vi "Steuerprogramm-29-05-17.vi"() -> ()   [LabVIEW 2010]
uses:
  Emil/Licor-Steuerung/HAGAR V/Licor-Steuerung/display/GUI_Cluster_sdv.ctl
  Emil/Licor-Steuerung/HAGAR V/Licor-Steuerung/display/GUI_Cluster_Parameter.ctl
  Emil/Licor-Steuerung/HAGAR V/Licor-Steuerung/control/Licor-Commands.ctl
  Emil/Licor-Steuerung/HAGAR V/Licor-Steuerung/control/Licor-Parameter.ctl
  Emil/Licor-Steuerung/LicorLI7000/conventions/Licor-Source.ctl
  Emil/Licor-Steuerung/HAGAR V/Licor-Steuerung/control/Licor-Pump.ctl
  Emil/Licor-Steuerung/HAGAR V/Licor-Steuerung/display/GUI_Cluster_Graph.ctl
  Emil/Licor-Steuerung/HAGAR V/Licor-Steuerung/control/Licor-Sequences.ctl
  <vilib>/rvi/interface/nirviMethod/nirviMethod.xnode
  C:/Users/HAGAR-IV/Desktop/Zeugs/markus/version feb 2012/FPGA Bitfiles/pertrasgcfpga2_FPGATarget_FPGA-Programm-01_A75D3647.lvbitx
  C:/Users/HAGAR-IV/Desktop/Zeugs/Johnny/pertrasgc fpga/FPGA-Programm-01-17.vi
  <vilib>/rvi/interface/common/niFpgaNodeNameForErrorReporting.ctl
  <vilib>/rvi/errors/niLvFpgaWhatHappensToTopLevelVI.ctl
  <vilib>/rvi/interface/nirviReadWriteControl/nirviReadWriteControl.xnode
  <vilib>/rvi/interface/nirviCloseFPGA/nirviCloseFPGA.xnode
  GVProbenvol.vi
  GVZeitenZyklen.vi
  GVECDs.vi
  GVZwangs.vi
  GVMethodenwechsel.vi
  GVTrapsMachs.vi
  GVHK1Hz.vi
  GVAIs.vi
  gvbooleschRT.vi
  GVMetavariablen.vi
  GVVentilposition.vi
  GVHorstSP.vi
  GVMWHorst.vi
  GVHeizenLH.vi
  <vilib>/Utility/error.llb/Error Cluster From Error Code.vi
  <vilib>/rvi/errors/niLvFpgaAdjustHostInterfaceError.vi
  GVaktuelleTDMS.vi
  Emil/Licor-Steuerung/HAGAR V/Licor-Steuerung/control/Emulate Licor output GV.vi
  GVChroms.vi
  GVZwangsMPV.vi
  <vilib>/FPGAPlugInAG/cRIO-9114/niLvFpga_Close_cRIO-9114.vi
  NiFpgaLv.dll
  Emil/Licor-Steuerung/HAGAR V/Licor-Steuerung/Licor-Steuerung.lvlib
  Emil/Licor-Steuerung/LicorLI7000/LicorLI7000.lvlib
panel:
  in  "Methode speichern":bool
  out "ZyklusNummernGesamt":i32[](array[numeric])
  in  "veränderte Methode benutzen":bool
  in  "Methode verändern":bool
  out "ZyklusNummern":i32[](array[numeric])
  out "Big Ben, Methodenzeit, Zykluszeit0, Zykluszeit1, Zykluszeit2A, Zykluszeit2B":i32[](array[numeric])
  in  "global stop RT":bool
  in  "Methode":i32(ring) items=["Bedingsmethode", "Startmethode", "Meßmodus", "Shut-up-Methode", "Test", "HAG2 1/2", "Startmethode", "HAG2 1/2 Aufwärmen", "LicorDruckProfil1", "LicorDruckProfil2", "LicorDruckProfil0", "LicorDruckProfil3"]
  in  "Registerkarte":T1(tab)
  out "SHOK?":bool[](array[boolean])
  out "schnelle Heizungen":string[](array[string])
  out "schnelle Heizungen":dbl[](array[numeric])
  out "HorstOK?":bool[](array[boolean])
  out "AIs3OK?":bool[](array[boolean])
  out "AIs1OK?":bool[](array[boolean])
  out "AIs1":dbl[](array[numeric])
  out "AIs1":string[](array[string])
  out "AIs2":string[](array[string])
  out "AIs3":string[](array[string])
  out "AIs2":dbl[](array[numeric])
  out "AIs3":dbl[](array[numeric])
  out "Metavariablen":string[](array[string])
  out "Metavariablen":dbl[](array[numeric])
  out "MWHorst":dbl[](array[numeric])
  out "HorstRegler":string[](array[string])
  out "AIs2OK?":bool[](array[boolean])
  out "Ventilposition":i32=1 min=1 max=6 step=1
  out "MVOK?":bool[](array[boolean])
  out "Housekeeping1":cluster{dbl[], dbl[]}(graph)
  in  "Zeitachse1":i32(ring)=1 items=["Zykluszeit [s] Mod0", "Zykluszeit [s] Mod1", "Zykluszeit [s] Mod2A", "Zykluszeit [s] Mod2B"]
  in  "dargestellte Größe 1":i32(ring)=1 items=["T1-Trap1 [°C]", "T1-Trap2 [°C]", "T1-StirlingKühlkopf [°C]", "T1-PreCol1 [°C]", "T1-PreCol2 [°C]", "T1-MainCol1a [°C]", "T1-MainCol1b [°C]", "T1-MainCol2a [°C]", "T1-MainCol2b [°C]", "T1-Bronkhorst1a [°C]", "T1-Bronkhorst1b [°C]", "T1-Bronkhorst2a [°C]", "T1-Bronkhorst2b [°C]", "T1-2Pos1B [°C]", "T1-Spare9", "T1-2Pos1A [°C]", "T1-Spare10", "T1-TurboPump [°C]", "T1-StirlingPlatine [°C]", "T1-Spare5", "T1-Spare6", "T1-Spare7", "T1-Spare8", "F1-MFM1", "F1-MFM0D [mL]", "P1-HeliumHP [bara]", "P1-HeliumLP [bara]", "P1-PumpVordruck [mbara]", "TurboSpeed", "I1-MS-AC [A]", "I1-Trap1 [A]", "I1-Trap2 [A]", "T2-ECD1a", "T2-ECD1b", "T2-ECD2a", "T2-ECD2b", "T2-Col1a", "T2-Col1b", "T2-Col2a", "T2-Col2b", "T2-Spare1", "T2-Spare2", "T2-Oven_a", "T2-Oven_b", "T2-Spare3", "T2-Spare4", "T2-Spare5", "F2-MFM0", "F2-MFM2A", "F2-MFM2B", "P2-N2O_HP", "P2-N2O_LP", "P2-CO2_HP", "P2-CO2_LP", "AI-Spare1", "FL-MFM1000mL", "AI-Spare3", "AI-Spare4", "StirlingAlarm", "StirlingEmerg.", "AI-Spare7", "AI-Spare8", "AI-Spare9", "FL-MFM30mL", "T0-DC/DC5", "I0-24V_M0", "I0-48V_M1", "I0-24V_M1", "I0-28V_M2", "T0-Spare3", "T0-Spare2", "T0-Spare4", "T0-DC/DC7", "I0-20V_Laptop", "I0-28V_M1", "I0-24V_M2", "I0-12V_Licor", "T0-Spare1", "T0-Drier", "T0-Spare5", "F0-MFM0A [L]", "TL-Licor_a", "P0-Span-HP", "P0-spare1", "P0-Stickstoff-LP", "P0-Helium-LP", "P0-Cal-HP", "P0-P9Tavco[bar]", "F0-MFM0B [L]", "TL-Licor_b", "P0-Span-LP", "P0-spare2", "P0-Stickstoff-HP", "P0-Helium-HP", "P0-Cal-LP", "F0-MFM3", "TemperaturTrap1[°C]", "TemperaturTrap2[°C]", "TemperaturPreMach1[°C]", "TemperaturPreMach2[°C]", "TemperaturMainMach1[°C]", "TemperaturMainMach2[°C]", "PrC0 [bara]", "PrC0-Licor [bara]", "PrC1-Säule1 [bara]", "PrC1-Säule2 [bara]", "MFC1-Sample [ml/min]", "PrC1-BackFlush1 [bara]", "PrC1-BackFlush2 [bara]", "MFC1-Reaktant [l/min]", "MFC2A[ml/min]", "MFC2B[ml/min]", "MFC2C[ul/min]", "PrC2A[bara]", "MFC2D[ml/min]", "MFC2E[ml/min]", "PrC2B[bara]"]
  out "Housekeeping2":cluster{dbl[], dbl[]}(graph)
  in  "Zeitachse2":i32(ring)=1 items=["Zykluszeit [s] Mod0", "Zykluszeit [s] Mod1", "Zykluszeit [s] Mod2A", "Zykluszeit [s] Mod2B"]
  in  "dargestellte Größe 2":i32(ring)=1 items=["T1-Trap1 [°C]", "T1-Trap2 [°C]", "T1-StirlingKühlkopf [°C]", "T1-PreCol1 [°C]", "T1-PreCol2 [°C]", "T1-MainCol1a [°C]", "T1-MainCol1b [°C]", "T1-MainCol2a [°C]", "T1-MainCol2b [°C]", "T1-Bronkhorst1a [°C]", "T1-Bronkhorst1b [°C]", "T1-Bronkhorst2a [°C]", "T1-Bronkhorst2b [°C]", "T1-2Pos1B [°C]", "T1-Spare9", "T1-2Pos1A [°C]", "T1-Spare10", "T1-TurboPump [°C]", "T1-StirlingPlatine [°C]", "T1-Spare5", "T1-Spare6", "T1-Spare7", "T1-Spare8", "F1-MFM1", "F1-MFM0D [mL]", "P1-HeliumHP [bara]", "P1-HeliumLP [bara]", "P1-PumpVordruck [mbara]", "TurboSpeed", "I1-MS-AC [A]", "I1-Trap1 [A]", "I1-Trap2 [A]", "T2-ECD1a", "T2-ECD1b", "T2-ECD2a", "T2-ECD2b", "T2-Col1a", "T2-Col1b", "T2-Col2a", "T2-Col2b", "T2-Spare1", "T2-Spare2", "T2-Oven_a", "T2-Oven_b", "T2-Spare3", "T2-Spare4", "T2-Spare5", "F2-MFM0", "F2-MFM2A", "F2-MFM2B", "P2-N2O_HP", "P2-N2O_LP", "P2-CO2_HP", "P2-CO2_LP", "AI-Spare1", "FL-MFM1000mL", "AI-Spare3", "AI-Spare4", "StirlingAlarm", "StirlingEmerg.", "AI-Spare7", "AI-Spare8", "AI-Spare9", "FL-MFM30mL", "T0-DC/DC5", "I0-24V_M0", "I0-48V_M1", "I0-24V_M1", "I0-28V_M2", "T0-Spare3", "T0-Spare2", "T0-Spare4", "T0-DC/DC7", "I0-20V_Laptop", "I0-28V_M1", "I0-24V_M2", "I0-12V_Licor", "T0-Spare1", "T0-Drier", "T0-Spare5", "F0-MFM0A [L]", "TL-Licor_a", "P0-Span-HP", "P0-spare1", "P0-Stickstoff-LP", "P0-Helium-LP", "P0-Cal-HP", "P0-P9Tavco[bar]", "F0-MFM0B [L]", "TL-Licor_b", "P0-Span-LP", "P0-spare2", "P0-Stickstoff-HP", "P0-Helium-HP", "P0-Cal-LP", "F0-MFM3", "TemperaturTrap1[°C]", "TemperaturTrap2[°C]", "TemperaturPreMach1[°C]", "TemperaturPreMach2[°C]", "TemperaturMainMach1[°C]", "TemperaturMainMach2[°C]", "PrC0 [bara]", "PrC0-Licor [bara]", "PrC1-Säule1 [bara]", "PrC1-Säule2 [bara]", "MFC1-Sample [ml/min]", "PrC1-BackFlush1 [bara]", "PrC1-BackFlush2 [bara]", "MFC1-Reaktant [l/min]", "MFC2A[ml/min]", "MFC2B[ml/min]", "MFC2C[ul/min]", "PrC2A[bara]", "MFC2D[ml/min]", "MFC2E[ml/min]", "PrC2B[bara]"]
  out "Detektor 2":cluster{dbl[], dbl[]}[](graph)
  in  "Detektor":i32(ring) items=["ECD1", "ECD2"]
  in  "HK1YMin":dbl
  in  "HK1YMax":dbl=100.0
  in  "HK2YMin":dbl
  in  "HK2YMax":dbl=100.0
  in  "DetYMin":dbl
  in  "DetYMax":dbl=100.0
  in  "NeuerRefstrom":bool
  in  "RefStromECD1":i16 min=0 max=2500 step=1
  in  "RefStromECD2":i16 min=0 max=2500 step=1
  out "schnelleAnzeige":cluster{dbl[], dbl[]}(graph)
  in  "TafelWischen!":bool
  in  "dargestellte Größe 3":i32(ring)=1 items=["TemperaturTrap1[°C]", "TemperaturTrap2[°C]", "TemperaturPreMach1[°C]", "TemperaturPreMach2[°C]", "TemperaturMainMach1[°C]", "TemperaturMainMach2[°C]", "PrC0 [bara]", "PrC0-Licor [bara]", "PrC1-Säule1 [bara]", "PrC1-Säule2 [bara]", "MFC1-Sample [ml/min]", "PrC1-BackFlush1 [bara]", "PrC1-BackFlush2 [bara]", "MFC1-Reaktant [l/min]", "MFC2A[ml/min]", "MFC2B[ml/min]", "MFC2C[ul/min]", "PrC2A[bara]", "MFC2D[ml/min]", "MFC2E[ml/min]", "PrC2B[bara]"]
  in  "An/Aus":bool
  in  "Registerkarte 2":T2(tab)
  in  "GUI_Cluster_Graph":T3={"time (global)"=0.0, "command queue"=[], "Rohdaten"=[], "Graph"={"X"=[], "Y"=[]}, "Manuelle Steuerung"={"Sequenz"=enum."test", "Manuelle Steuerung An/Aus"=FALSE}, "Sequenz out"={"sequence"=enum."WAIT", "Zeitpunkt next"=0.0, "delta t"=0.0}} caption="Cluster" {"Sequenz out"."Zeitpunkt next" format="%<%H:%M:%S%3u>T"; "time (global)" format="%<%H:%M:%S%3u\n%m/%d/%y>T"}
  in  "GUI_Cluster_Parameter":T5={"warmup (sequence)"=[{"time"=60, "Enum"=enum."wait"}], "calibrate S (sequence)"=[{"time"=60, "Enum"=enum."wait"}, {"time"=2, "Enum"=enum."getCalibrationParameter"}, {"time"=8, "Enum"=enum."calibration-S-CO2"}, {"time"=2, "Enum"=enum."getCalibrationParameter"}], "calibrate Z (sequence)"=[{"time"=60, "Enum"=enum."wait"}, {"time"=2, "Enum"=enum."getCalibrationParameter"}, {"time"=8, "Enum"=enum."calibration-Z-H2O"}, {"time"=2, "Enum"=enum."getCalibrationParameter"}, {"time"=8, "Enum"=enum."calibration-Z-CO2"}, {"time"=2, "Enum"=enum."getCalibrationParameter"}], "initialize (sequence)"=[{"time"=30, "Enum"=enum."wait"}, {"time"=2, "Enum"=enum."setPumpSlow"}, {"time"=2, "Enum"=enum."setPumpMedium"}, {"time"=2, "Enum"=enum."setPumpFast"}, {"time"=10, "Enum"=enum."initialize"}, {"time"=4, "Enum"=enum."getCalibrationParameter"}, {"time"=2, "Enum"=enum."resetH2O"}, {"time"=4, "Enum"=enum."resetCO2"}, {"time"=4, "Enum"=enum."getCalibrationParameter"}, {"time"=2, "Enum"=enum."setZeroParameter"}, {"time"=4, "Enum"=enum."getCalibrationParameter"}, {"time"=2, "Enum"=enum."setReference"}, {"time"=4, "Enum"=enum."getLicorTime"}, {"time"=5, "Enum"=enum."getInfo"}], "Licor-parameter"={"CO2 ref"=402.3, "CO2 span"=392.3, "H2O ref"=0.0, "H2O span"=0.0, "Zi"=1.2, "Zt"=6.494e-05, "Zm"=0.0, "S"=1.34, "Temp [C]"=45.0, "Pressure [hPa]"=1013.0, "Licor-Sources"=["CO2A W", "CO2B W", "H2OA W", "H2OB W", "T C", "T V", "P kPa", "P V", "RH %", "CO2A um/m", "CO2B um/m", "H2OA mm/m", "H2OB mm/m"], "Licor-Pump"="Off", "Zeitstempel"=timestamp(0 s since 1904-01-01)}} {"Licor-parameter"."Pressure [hPa]" format="%_5g"; "Licor-parameter"."Temp [C]" format="%.2f"; "Licor-parameter"."CO2 ref" format="%.2f"; "Licor-parameter"."CO2 span" format="%.2g"; "Licor-parameter"."H2O ref" format="%.2g"; "Licor-parameter"."H2O span" format="%.2g"; "Licor-parameter"."Zt" format="%#_4g"}
  in  "GUI_Cluster_sdv":T10={"Graph_sdv"={"X"=[], "Y"=[]}, "Breite"=20, "Berechnen"=FALSE, "residue"=0.0} {"residue" format="%_6g"}
  in  "VISA resource name":refnum<visa-resource-name>="ASRL1::INSTR" caption="VISA-Ressourcenname"
  in  "ServosWarmHigh (us)KaltHigh(us)":T11={"Servo1WarmHigh(us)"=1000, "Servo1KaltHigh(us)"=1000, "Servo2WarmHigh(us)"=2030, "Servo2KaltHigh(us)"=2030}
  out "TDMSwriteECD":errorcluster
  out "AIsFIFOread":errorcluster
  out "MWTrapsMachs":errorcluster
  out "TDMSwriteHK":errorcluster
  out "TDMScloseHK":errorcluster
  out "TDMSopenHK":errorcluster
  out "TDMScloseECD2":errorcluster
  out "TDMSopenECD2":errorcluster
  out "TDMScloseECD1":errorcluster
  out "TDMSopenECD1":errorcluster
  out "FIFOwriteRS485":errorcluster
  out "SerielleKomm.":errorcluster
  out "LH":errorcluster
  out "Zyklus":errorcluster
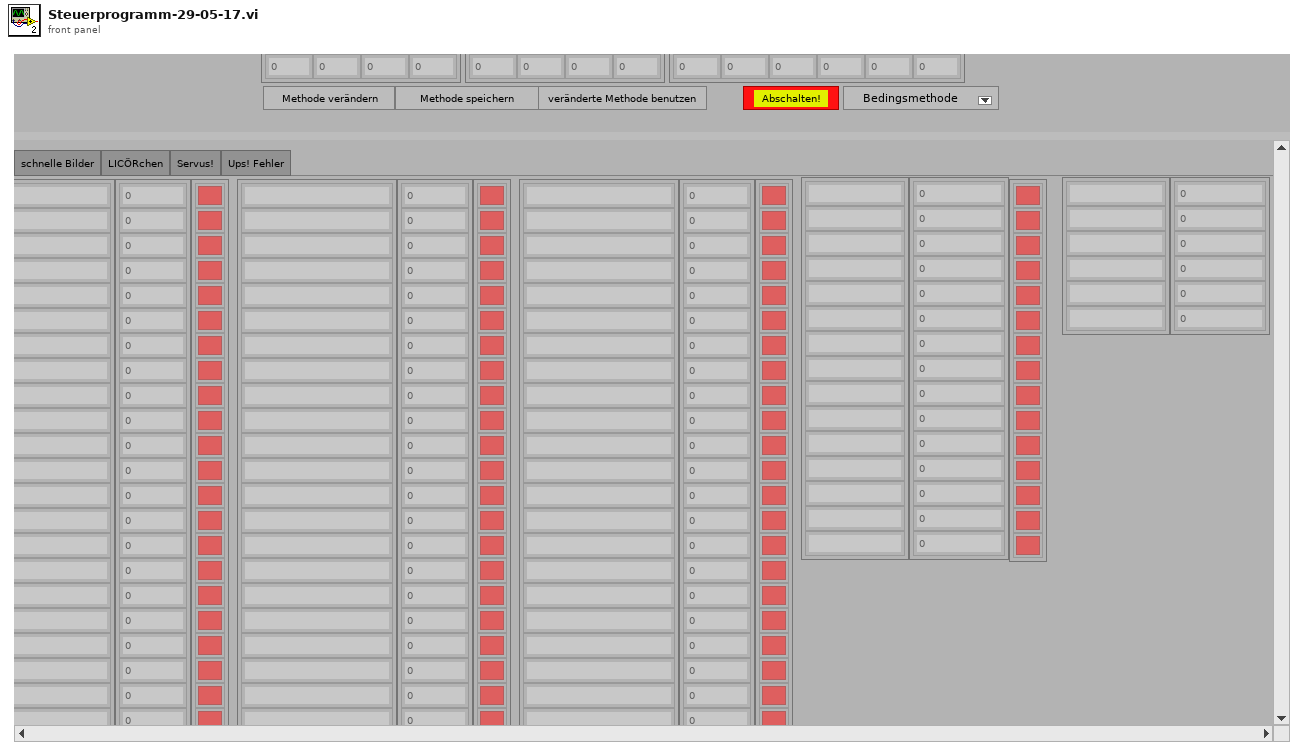
[diagram p1: front panel]
types:
  T1 = enum32{"Tabellen", "Bilder", "schnelle Bilder", "LICÖRchen", "Servus!", "Ups! Fehler"}
  T2 = enum32{"Graph", "Parameter / Sequenzen", "sdv", "debug"}
  T3 = typedef "Licor-Steuerung.lvlib/GUI_Cluster_Graph.ctl" = cluster{"time (global)":dbl, "command queue":cluster{"Zeit [s]":i32, "Befehl":string}[], "Rohdaten":string[], "Graph":cluster{"X":dbl[], "Y":dbl[]}, "Manuelle Steuerung":cluster{"Sequenz":T4, "Manuelle Steuerung An/Aus":bool}, "Sequenz out":cluster{"sequence":T4, "Zeitpunkt next":dbl, "delta t":dbl}}
  T4 = typedef "Licor-Steuerung.lvlib/Licor-Sequences.ctl" = enum16{"test", "WAIT", "warmup", "initialize", "calibrate Z", "calibrate S"}
  T5 = typedef "Licor-Steuerung.lvlib/GUI_Cluster_Parameter.ctl" = cluster{"warmup (sequence)":cluster{"time":i32, "Enum":T6}[], "calibrate S (sequence)":cluster{"time":i32, "Enum":T6}[], "calibrate Z (sequence)":cluster{"time":i32, "Enum":T6}[], "initialize (sequence)":cluster{"time":i32, "Enum":T6}[], "Licor-parameter":T7}
  T6 = typedef "Licor-Steuerung.lvlib/Licor-Commands.ctl" = enum16{"wait", "initialize", "resetCO2", "resetH2O", "getReference", "setReference", "calibration-Z-CO2", "calibration-Z-H2O", "calibration-S-CO2", "calibration-S-H2O", "getCalibrationParameter", "setZeroParameter", "setLicorTime", "getLicorTime", "setPumpFlowrate", "setPumpSlow", "setPumpMedium", "setPumpFast", "getInfo"}
  T7 = typedef "Licor-Steuerung.lvlib/Licor-Parameter.ctl" = cluster{"CO2 ref":dbl, "CO2 span":dbl, "H2O ref":dbl, "H2O span":dbl, "Zi":dbl, "Zt":dbl, "Zm":dbl, "S":dbl, "Temp [C]":dbl, "Pressure [hPa]":dbl, "Licor-Sources":T8[], "Licor-Pump":T9, "Zeitstempel":timestamp}
  T8 = typedef "LicorLI7000.lvlib/Licor-Source.ctl" = string
  T9 = typedef "Licor-Steuerung.lvlib/Licor-Pump.ctl" = string
  T10 = typedef "Licor-Steuerung.lvlib/GUI_Cluster_sdv.ctl" = cluster{"Graph_sdv":cluster{"X":dbl[], "Y":dbl[]}, "Breite":i32, "Berechnen":bool, "residue":dbl}
  T11 = cluster{"Servo1WarmHigh(us)":u32, "Servo1KaltHigh(us)":u32, "Servo2WarmHigh(us)":u32, "Servo2KaltHigh(us)":u32}
  T12 = cluster{"DIOsMod0Nr":i32[], "DIOsMod1Nr":i32[], "DIOsMod2ANr":i32[], "DIOsMod2BNr":i32[], "AIsLH":i32[], "AnzahlRegler/Modul":i32[], "Regler für den Probenfluß":i32, "SPvorgebenMod0":string[], "SPvorgebenMod1":string[], "SPvorgebenMod2A":string[], "SPvorgebenMod2B":string[], "MWAntwortMod0":string[], "MWAntwortMod1":string[], "MWAntwortMod2A":string[], "MWAntwortMod2B":string[], "FaktorMod0":dbl[], "FaktorMod1":dbl[], "FaktorMod2A":dbl[], "FaktorMod2B":dbl[], "MWabfragenMod0":string[], "MWabfragenMod1":string[], "MWabfragenMod2A":string[], "MWabfragenMod2B":string[], "Modul1/AI koeff":dbl[][], "Modul2/AI koeff":dbl[][], "Modul3/AI koeff":dbl[][], "Traps/MachsKoeff":dbl[][], "Modul1/AIsNamen":string[], "Modul2/AIsNamen":string[], "Modul3/AIsNamen":string[], "DIOsMod0Name":string[], "DIOsMod1Name":string[], "DIOsMod2AName":string[], "DIOsMod2BName":string[], "ReglerNameMod0":string[], "ReglerNameMod1":string[], "ReglerNameMod2A":string[], "ReglerNameMod2B":string[], "Startmethode":i32, "Dateiordner Housekeeping":path, "Dateiname Housekeeping":string, "DateiordnerECD1":path, "DateinameECD1":string, "DateiordnerECD2":path, "DateinameECD2":string, "LangsameHeizungen":string[], "ModuleLH":i32[], "Metavariablen":string[], "Modul1/AI sicherer Bereich":dbl[][], "Modul2/AI sicherer Bereich":dbl[][], "Modul3/AI sicherer Bereich":dbl[][], "Traps/Machs sicherer Bereich":dbl[][], "ReglerMod0 sicherer Bereich":dbl[][], "ReglerMod1 sicherer Bereich":dbl[][], "ReglerMod2A sicherer Bereich":dbl[][], "ReglerMod2B sicherer Bereich":dbl[][], "Metavariablen grüner Bereich":dbl[][]}
  T13 = cluster{"Zykluslängen [s]":dbl[], "ZeitpktDIOsMod0":dbl[], "ZeitpktDIOsMod1":dbl[], "ZeitpktDIOsMod2A":dbl[], "ZeitpktDIOsMod2B":dbl[], "DIOsSPMod0":bool[][], "DIOsSPMod1":bool[][], "DIOsSPMod2A":bool[][], "DIOsSPMod2B":bool[][], "Mod0HorstZeitpkt":dbl[], "Mod1HorstZeitpkt":dbl[], "Mod2AHorstZeitpkt":dbl[], "Mod2BHorstZeitpkt":dbl[], "HorstSPMod0":dbl[][], "HorstSPMod1":dbl[][], "HorstSPMod2A":dbl[][], "HorstSPMod2B":dbl[][], "LHSetpoints":dbl[], "LHHeizen?":bool[], "ZPktFPGABoolesch":dbl[], "FPGABoolesch":bool[][], "ZeitpktFPGAPID":dbl[], "FPGAPID":cluster{"proportional gain (Kc)":fxp<+/-,16,8>, "integral gain (Kc*Ts/Ti)":fxp<+/-,16,8>, "derivative gain (Kc*Td/Ts)":fxp<+/-,16,8>}[][], "ZeitpktFPGAFixp":dbl[], "SHSetpoints":dbl[][], "t_PreMach1":dbl[], "T_PreMach1":dbl[], "t_PreMach2":dbl[], "T_PreMach2":dbl[], "PIDs für \"träge\" Heizungen":cluster{"proportional gain (Kc)":dbl, "integral time (Ti, min)":dbl, "derivative time (Td, min)":dbl}[], "Zwangsbedingungen":dbl[][], "Dateien fürs MS schicken?":bool, "ZeitpunkteMPV":dbl[], "SPMPV":i32[], "ZeitpktMS-1":dbl, "ZeitpktMS-2":dbl, "Int.Start1":dbl, "Int.Stop1":dbl, "Int.Start2":dbl, "Int.Stop2":dbl, "Methodenname":string, "t_MainMach1":dbl[], "T_MainMach1":dbl[], "t_MainMach2":dbl[], "T_MainMach2":dbl[]}[]
  T14 = enum16{"open", "replace", "create", "open or create", "replace or create", "replace or create with confirmation"}
  T15 = typedef "niFpgaNodeNameForErrorReporting.ctl" = enum16{"Open FPGA VI Reference", "Read/Write Control", "Invoke Method: Abort", "Invoke Method: Acknowledge IRQ", "Invoke Method: Download", "Invoke Method: FIFO.Configure", "Invoke Method: FIFO.Read", "Invoke Method: FIFO.Start", "Invoke Method: FIFO.Stop", "Invoke Method: FIFO.Write", "Invoke Method: Reset", "Invoke Method: Run", "Invoke Method: Wait on IRQ", "Close FPGA VI Reference"}
  T16 = typedef "niLvFpgaWhatHappensToTopLevelVI.ctl" = enum16{"top level VI scripted behind XNode", "top level VI inlined behind XNode"}
  T17 = cluster{"Zyklus1":i32, "Zeitachse1":i32, "dargestellte Größe 1":i32, "Zyklus2":i32, "Zeitachse2":i32, "dargestellte Größe 2":i32}
  T18 = cluster{"DIOsMod0Name":string[], "DIOsMod1Name":string[], "DIOsMod2AName":string[], "DIOsMod2BName":string[], "ReglerNameMod0":string[], "ReglerNameMod1":string[], "ReglerNameMod2A":string[], "ReglerNameMod2B":string[], "LangsameHeizungen":string[]}
  T19 = cluster{"Zykluslängen [s]":dbl[], "ZeitpktDIOsMod0":dbl[], "ZeitpktDIOsMod1":dbl[], "ZeitpktDIOsMod2A":dbl[], "ZeitpktDIOsMod2B":dbl[], "DIOsSPMod0":bool[][], "DIOsSPMod1":bool[][], "DIOsSPMod2A":bool[][], "DIOsSPMod2B":bool[][], "Mod0HorstZeitpkt":dbl[], "Mod1HorstZeitpkt":dbl[], "Mod2AHorstZeitpkt":dbl[], "Mod2BHorstZeitpkt":dbl[], "HorstSPMod0":dbl[][], "HorstSPMod1":dbl[][], "HorstSPMod2A":dbl[][], "HorstSPMod2B":dbl[][], "LHSetpoints":dbl[], "LHHeizen?":bool[], "ZPktFPGABoolesch":dbl[], "FPGABoolesch":bool[][], "ZeitpktFPGAPID":dbl[], "FPGAPID":cluster{"proportional gain (Kc)":fxp<+/-,16,8>, "integral gain (Kc*Ts/Ti)":fxp<+/-,16,8>, "derivative gain (Kc*Td/Ts)":fxp<+/-,16,8>}[][], "ZeitpktFPGAFixp":dbl[], "SHSetpoints":dbl[][], "t_PreMach1":dbl[], "T_PreMach1":dbl[], "t_PreMach2":dbl[], "T_PreMach2":dbl[], "PIDs für \"träge\" Heizungen":cluster{"proportional gain (Kc)":dbl, "integral time (Ti, min)":dbl, "derivative time (Td, min)":dbl}[], "Zwangsbedingungen":dbl[][], "Dateien fürs MS schicken?":bool, "ZeitpunkteMPV":dbl[], "SPMPV":i32[], "ZeitpktMS-1":dbl, "ZeitpktMS-2":dbl, "Int.Start1":dbl, "Int.Stop1":dbl, "Int.Start2":dbl, "Int.Stop2":dbl, "Methodenname":string, "t_MainMach1":dbl[], "T_MainMach1":dbl[], "t_MainMach2":dbl[], "T_MainMach2":dbl[]}
  T20 = cluster{"Modul1/AI sicherer Bereich":dbl[][], "Modul2/AI sicherer Bereich":dbl[][], "Modul3/AI sicherer Bereich":dbl[][], "Traps/Machs sicherer Bereich":dbl[][], dbl[][], "Metavariablen grüner Bereich":dbl[][]}
  T21 = cluster{"created path":path, "created path":path, "created path":path, "Dateiname Housekeeping":string, "DateinameECD1":string, "DateinameECD2":string, "tdms0":refnum<k34>, "tdms1":refnum<k34>, "tdms0":refnum<k34>, "tdms1":refnum<k34>, "tdms0":refnum<k34>, "tdms1":refnum<k34>}
  T22 = cluster{"proportional gain (Kc)":fxp<+/-,16,8>, "integral gain (Kc*Ts/Ti)":fxp<+/-,16,8>, "derivative gain (Kc*Td/Ts)":fxp<+/-,16,8>}[][]
  T23 = cluster{"proportional gain (Kc)":dbl, "integral time (Ti, min)":dbl, "derivative time (Td, min)":dbl}[]
  T24 = cluster{cluster{"ZeitpktDIOsMod2B":dbl[]}[], cluster{"DIOsSPMod2B":bool[][]}[], cluster{"Mod2BHorstZeitpkt":dbl[]}[], cluster{"HorstSPMod2B":dbl[][]}[], "LHHeizen?":bool[], "ZPktFPGABoolesch":dbl[], "FPGABoolesch":bool[][], "ZeitpktFPGAPID":dbl[], "FPGAPID":cluster{"proportional gain (Kc)":fxp<+/-,16,8>, "integral gain (Kc*Ts/Ti)":fxp<+/-,16,8>, "derivative gain (Kc*Td/Ts)":fxp<+/-,16,8>}[][], "ZeitpktFPGAFixp":dbl[], "SHSetpoints":dbl[][], "t_PreMach1":dbl[], "T_PreMach1":dbl[], "t_PreMach2":dbl[], "T_PreMach2":dbl[], "ZeitpunkteMPV":dbl[], "SPMPV":i32[], "t_MainMach1":dbl[], "T_MainMach1":dbl[], "t_MainMach2":dbl[], "T_MainMach2":dbl[]}
  T25 = cluster{"Zykluslängen [s]":dbl[], "ZeitpktDIOsMod0":dbl[], "ZeitpktDIOsMod1":dbl[], "ZeitpktDIOsMod2A":dbl[], "ZeitpktDIOsMod2B":dbl[], "DIOsSPMod0":bool[][], "DIOsSPMod1":bool[][], "DIOsSPMod2A":bool[][], "DIOsSPMod2B":bool[][], "Mod0HorstZeitpkt":dbl[], "Mod1HorstZeitpkt":dbl[], "Mod2AHorstZeitpkt":dbl[], "Mod2BHorstZeitpkt":dbl[], "HorstSPMod0":dbl[][], "HorstSPMod1":dbl[][], "HorstSPMod2A":dbl[][], "HorstSPMod2B":dbl[][], "LangsameHeizungenSP":dbl[], "LHHeizen?":bool[], "ZPktFPGABoolesch":dbl[], "FPGABoolesch":bool[][], "ZeitpktFPGAPID":dbl[], "FPGAPID":cluster{"proportional gain (Kc)":fxp<+/-,16,8>, "integral gain (Kc*Ts/Ti)":fxp<+/-,16,8>, "derivative gain (Kc*Td/Ts)":fxp<+/-,16,8>}[][], "ZeitpktFPGAFixp":dbl[], "FPGAFixp":dbl[][], "t_PreMach1":dbl[], "T_PreMach1":dbl[], "t_PreMach2":dbl[], "T_PreMach2":dbl[], "PIDs für \"träge\" Heizungen":cluster{"proportional gain (Kc)":dbl, "integral time (Ti, min)":dbl, "derivative time (Td, min)":dbl}[], "Zwangsbedingungen":dbl[][], "MS-Daten?":bool, "ZeitpunkteMPV":dbl[], "SetpointMPV":i32[], "ZeitpktMS-1":dbl, "ZeitpktMS-2":dbl, "Int.Start1":dbl, "Int.Stop1":dbl, "Int.Start2":dbl, "Int.Stop2":dbl, "Methodenname":string, "t_MainMach1":dbl[], "T_MainMach1":dbl[], "t_MainMach2":dbl[], "T_MainMach2":dbl[]}
  T26 = cluster{"ZyklusNummern":i32[], "ZeilennummernDIOs":i32[], "ZwangsDIO?":cluster{bool[]}[], "ZeilennummernHorst":i32[], "ZwangsHorst?":cluster{bool[]}[], "ZeileFPGABoolesch":i32, "ZwangsFPGABoolesch?":bool[], "ZeileFPGAPID":i32, "ZeileFPGAFixp":i32, "ZeilePreMach1":i32, "ZeilePreMach2":i32, "ZeilennummerMPV":i32, "ZeileMainMach1":i32, "ZeileMainMach2":i32, "ZwangsMPV?":bool}
  T27 = cluster{"ZyklusNummern":i32[], i32[], "ZwangsDIO?":cluster{bool[]}[], i32[], "ZwangsHorst?":cluster{bool[]}[], i32, "ZwangsFPGABoolesch?":bool[], i32, i32, "ZeileMach":i32, "ZeileMach":i32, i32, "ZeileMach":i32, "ZeileMach":i32, "ZwangsMPV?":bool}
  T28 = cluster{string[], string[], string[], dbl[], dbl[], dbl[]}
  T29 = cluster{"Befehle1":string[], "Befehle2":string[], "Befehle3":string[]}
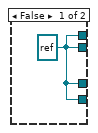
[diagram p2: hidden frame]
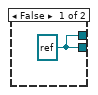
[diagram p3: hidden frame]
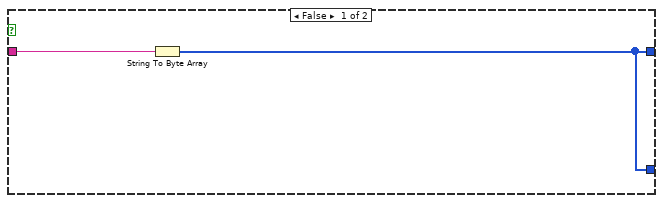
[diagram p6: hidden frame]
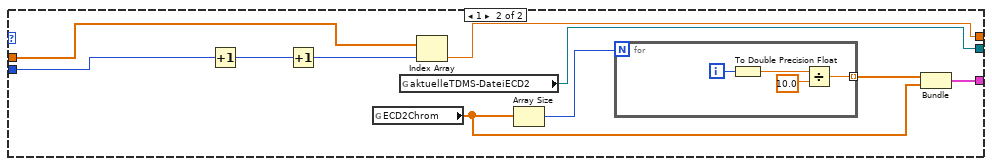
[diagram p13: hidden frame]
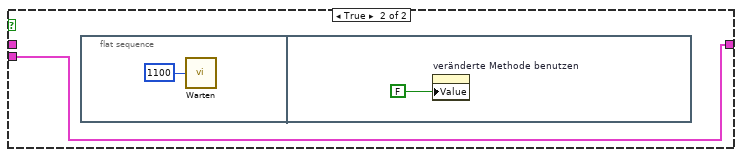
[diagram p14: hidden frame]
diagram:
  n1 = Open/Create/Replace File(file path (use dialog)=path "c:/einstellungen.perx" ("Datei (Dialog verwenden)"), operation (0:open)=T14."open" ("Operation (0:Öffnen)")) -> (refnum out=w13:refnum<file>)  [unwired: 4 in, 2 out]
  n2 = Open/Create/Replace File(file path (use dialog)=path "c:/methoden.per" ("Datei (Dialog verwenden)"), operation (0:open)=T14."open" ("Operation (0:Öffnen)")) -> (refnum out=w8:refnum<file>)  [unwired: 4 in, 2 out]
  n3 = Read from Binary File(5:T12 {"DIOsMod0Nr"=[], "DIOsMod1Nr"=[], "DIOsMod2ANr"=[], "DIOsMod2BNr"=[], "AIsLH"=[], "AnzahlRegler/Modul"=[], "Regler für den Probenfluß"=0, "SPvorgebenMod0"=[], "SPvorgebenMod1"=[], "SPvorgebenMod2A"=[], "SPvorgebenMod2B"=[], "MWAntwortMod0"=[], "MWAntwortMod1"=[], "MWAntwortMod2A"=[], "MWAntwortMod2B"=[], "FaktorMod0"=[], "FaktorMod1"=[], "FaktorMod2A"=[], "FaktorMod2B"=[], "MWabfragenMod0"=[], "MWabfragenMod1"=[], "MWabfragenMod2A"=[], "MWabfragenMod2B"=[], "Modul1/AI koeff"=[], "Modul2/AI koeff"=[], "Modul3/AI koeff"=[], "Traps/MachsKoeff"=[], "Modul1/AIsNamen"=[], "Modul2/AIsNamen"=[], "Modul3/AIsNamen"=[], "DIOsMod0Name"=[], "DIOsMod1Name"=[], "DIOsMod2AName"=[], "DIOsMod2BName"=[], "ReglerNameMod0"=[], "ReglerNameMod1"=[], "ReglerNameMod2A"=[], "ReglerNameMod2B"=[], "Startmethode"=0, "Dateiordner Housekeeping"=path "", "Dateiname Housekeeping"="", "DateiordnerECD1"=path "", "DateinameECD1"="", "DateiordnerECD2"=path "", "DateinameECD2"="", "LangsameHeizungen"=[], "ModuleLH"=[], "Metavariablen"=[], "Modul1/AI sicherer Bereich"=[], "Modul2/AI sicherer Bereich"=[], "Modul3/AI sicherer Bereich"=[], "Traps/Machs sicherer Bereich"=[], "ReglerMod0 sicherer Bereich"=[], "ReglerMod1 sicherer Bereich"=[], "ReglerMod2A sicherer Bereich"=[], "ReglerMod2B sicherer Bereich"=[], "Metavariablen grüner Bereich"=[]} ("output cluster"), 11:w13) -> (2:w11:T12, 3:w12:refnum<file>)  [unwired: 4 in, 2 out]
  n4 = Read from Binary File(5:T13 [], 11:w8) -> (2:w6:T13, 3:w7:refnum<file>)  [unwired: 4 in, 2 out]
  n5 = Close File(refnum=w12) -> ()  [unwired: 1 in, 2 out]
  n6 = Close File(refnum=w7) -> ()  [unwired: 1 in, 2 out]
  n7 = flat-sequence {
    tunnel: [w55] -> w41
    tunnel: [w112] -> w40
    tunnel: [w59] -> w38
    tunnel: [w246] -> w37
    tunnel: [w248] -> w36
    tunnel: [w240] -> w35
    tunnel: [w247] -> w34
    tunnel: [w170] -> w33
    tunnel: [w239] -> w32
    tunnel: [w238] -> w31
    tunnel: [w232] -> w30
    tunnel: [w173] -> w29
    tunnel: [w147] -> w28
    tunnel: [w245] -> w27
    tunnel: [w237] -> w26
    tunnel: [w236] -> w25
    tunnel: [w228] -> w24
    tunnel: [w227] -> w23
    tunnel: [w226] -> w22
    tunnel: [w225] -> w21
    tunnel: [w224] -> w20
    tunnel: [w223] -> w19
    tunnel: [w220] -> w18
    tunnel: [w202] -> w17
    tunnel: w11 -> [w88]
    tunnel: [w201] -> w16
    tunnel: w6 -> [w113]
    tunnel: [w112] -> w5
    tunnel: [w88] -> w3
    tunnel: [w50] -> w1
    tunnel: w41 -> [w445]
    tunnel: w40 -> [w518]
    tunnel: [w445] -> w39
    tunnel: w38 -> [_]
    tunnel: w37 -> [w476]
    tunnel: w36 -> [w475]
    tunnel: w35 -> [w477]
    tunnel: w34 -> [w474]
    tunnel: w33 -> [w449]
    tunnel: w32 -> [w444]
    tunnel: w31 -> [w441]
    tunnel: w30 -> [w438]
    tunnel: w29 -> [w439]
    tunnel: w28 -> [w442]
    tunnel: w27 -> [w516]
    tunnel: w26 -> [w447]
    tunnel: w25 -> [w517]
    tunnel: w24 -> [w420]
    tunnel: w23 -> [w419]
    tunnel: w22 -> [w418]
    tunnel: w21 -> [w514]
    tunnel: w20 -> [w513]
    tunnel: w19 -> [w512]
    tunnel: w18 -> [w466]
    tunnel: w17 -> [w448]
    tunnel: w16 -> [w437]
    tunnel: w6 -> [w436]
    tunnel: w5 -> [w434]
    tunnel: w3 -> [_]
    tunnel: w1 -> [w413]
    tunnel: w39 -> [w1355]
    frame #0 {
      w114 = TRUE
      w129 = 0.0 ("Probenvol.1")
      w136 = dbl[] [-1.0] ("ECD1MW")
      w137 = FALSE ("ECD1Empfangen?")
      w128 = string[] ["TemperaturTrap1[°C]", "TemperaturTrap2[°C]", "TemperaturPreMach1[°C]", "TemperaturPreMach2[°C]", "TemperaturMainMach1[°C]", "TemperaturMainMach2[°C]"]
      w243 = string[] ["Big Ben [s]", "Methodenzeit [s]", "Zykluszeit [s] Mod0", "Zykluszeit [s] Mod1", "Zykluszeit [s] Mod2A", "Zykluszeit [s] Mod2B"]
      w233 = FALSE ("Undefinierte Werte möglich")
      w234 = FALSE ("global stop RT")
      n8 = for {
        tunnel: [w408] -> w241 mode=indexing
        tunnel: w113 -> [w409] mode=indexing
        n9 = Unbundle(w409) -> ("Methodenname"=w408:string)  [unwired: 44 out]
      }
      n10 = Unbundle(w88) -> ("DIOsMod0Nr"=w157:i32[], "DIOsMod1Nr"=w156:i32[], "DIOsMod2ANr"=w155:i32[], "DIOsMod2BNr"=w154:i32[], "AIsLH"=w144:i32[], "AnzahlRegler/Modul"=w147:i32[], "Regler für den Probenfluß"=w201:i32, "SPvorgebenMod0"=w200:string[], "SPvorgebenMod1"=w199:string[], "SPvorgebenMod2A"=w198:string[], "SPvorgebenMod2B"=w197:string[], "MWAntwortMod0"=w196:string[], "MWAntwortMod1"=w195:string[], "MWAntwortMod2A"=w194:string[], "MWAntwortMod2B"=w193:string[], "FaktorMod0"=w192:dbl[], "FaktorMod1"=w191:dbl[], "FaktorMod2A"=w190:dbl[], "FaktorMod2B"=w189:dbl[], "MWabfragenMod0"=w188:string[], "MWabfragenMod1"=w187:string[], "MWabfragenMod2A"=w186:string[], "MWabfragenMod2B"=w185:string[], "Modul1/AI koeff"=w184:dbl[][], "Modul2/AI koeff"=w183:dbl[][], "Modul3/AI koeff"=w182:dbl[][], "Traps/MachsKoeff"=w181:dbl[][], "Modul1/AIsNamen"=w180:string[], "Modul2/AIsNamen"=w179:string[], "Modul3/AIsNamen"=w178:string[], "DIOsMod0Name"=w86:string[], "DIOsMod1Name"=w87:string[], "DIOsMod2AName"=w85:string[], "DIOsMod2BName"=w84:string[], "ReglerNameMod0"=w103:string[], "ReglerNameMod1"=w102:string[], "ReglerNameMod2A"=w101:string[], "ReglerNameMod2B"=w100:string[], "Startmethode"=w112:i32, "Dateiordner Housekeeping"=w83:path, "Dateiname Housekeeping"=w177:string, "DateiordnerECD1"=w97:path, "DateinameECD1"=w176:string, "DateiordnerECD2"=w96:path, "DateinameECD2"=w175:string, "LangsameHeizungen"=w174:string[], "ModuleLH"=w169:i32[], "Metavariablen"=w107:string[], "Modul1/AI sicherer Bereich"=w54:dbl[][], "Modul2/AI sicherer Bereich"=w53:dbl[][], "Modul3/AI sicherer Bereich"=w52:dbl[][], "Traps/Machs sicherer Bereich"=w51:dbl[][], "ReglerMod0 sicherer Bereich"=w49:dbl[][], "ReglerMod1 sicherer Bereich"=w48:dbl[][], "ReglerMod2A sicherer Bereich"=w47:dbl[][], "ReglerMod2B sicherer Bereich"=w46:dbl[][], "Metavariablen grüner Bereich"=w44:dbl[][])
      "Metavariablen" <- w107
      n11 = Initialize Array(0, 4 ("Dimension")) -> (w130:i32[])
      n12 = Initialize Array(0.0 ("Element"), 6 ("Dimension")) -> (w133:dbl[])
      n13 = global write "GVMethodenwechsel.vi" "Methodenwechsel?"(FALSE ("Methodenwechsel?")) -> ()
      n14 = local write "NeuerRefstrom"(FALSE ("NeuerRefstrom")) -> ()
      n15 = global write "GVProbenvol.vi" "Probenvol.1"(w129) -> ()
      n16 = global write "GVProbenvol.vi" "Probenvol.2"(w129) -> ()
      n17 = global write "GVECDs.vi" "ECD1MW"(w136) -> ()
      n18 = global write "GVECDs.vi" "ECD2MW"(w136) -> ()
      n19 = global write "GVECDs.vi" "ECD1Empfangen?"(w137) -> ()
      n20 = global write "GVECDs.vi" "ECD2Empfangen?"(w137) -> ()
      n21 = property on="dargestellte Größe 2" class="Ring (strict)"("AllowUndefVals"=w233) -> ()  [unwired: 2 in, 2 out]
      n22 = property on="Zeitachse2" class="Ring (strict)"("AllowUndefVals"=w233) -> ()  [unwired: 2 in, 2 out]
      n23 = property on="Zeitachse1" class="Ring (strict)"("AllowUndefVals"=w233) -> ()  [unwired: 2 in, 2 out]
      n24 = property on="dargestellte Größe 1" class="Ring (strict)"("AllowUndefVals"=w233) -> ()  [unwired: 2 in, 2 out]
      n25 = property on="Methode" class="Ring (strict)"("AllowUndefVals"=w233) -> ()  [unwired: 2 in, 2 out]
      n26 = local write "global stop RT"(w234) -> ()
      n27 = global write "gvbooleschRT.vi" "global stop RT"(w234) -> ()
      n28 = global write "GVZeitenZyklen.vi" "ZyklusNummern"(w130) -> ()
      n29 = global write "GVZeitenZyklen.vi" "ZyklusNummernGesamt"(w130) -> ()
      n30 = global write "GVZeitenZyklen.vi" "Big Ben, Methodenzeit, Zykluszeit0, Zykluszeit1, Zykluszeit2A, Zykluszeit2B"(w133) -> ()
      n31 = property on="Methode" class="Ring (strict)"("Value"=w112) -> ()  [unwired: 2 in, 2 out]
      n32 = Initialize Array(-1.0 ("Element"), 6 ("Dimension")) -> (w140:dbl[])
      n33 = Initialize Array(FALSE, 10 ("Dimension")) -> (w148:bool[])
      n34 = Initialize Array(-1.0 ("Element"), 96 ("Dimension")) -> (w141:dbl[])
      n35 = global write "GVZwangs.vi" "ZwangsFPGABoolesch!"(w148) -> ()
      n36 = global write "GVZwangs.vi" "ZwangsFPGABoolesch?"(w148) -> ()
      n37 = global write "GVTrapsMachs.vi" "Traps/Machs"(w140) -> ()
      n38 = global write "GVAIs.vi" "AIs"(w141) -> ()
      n39 = for {
        tunnel: w147 -> [w386] mode=indexing
        tunnel: [w383] -> w146 mode=indexing
        tunnel: [w381] -> w145 mode=indexing
        n40 = Initialize Array(0.0 ("Element"), w386) -> (w384:dbl[])
        n41 = Initialize Array(FALSE, w386) -> (w382:bool[])
        n42 = Bundle(w384) -> (w383:cluster{dbl[]})  [unwired: 1 in]
        n43 = Bundle(w382) -> (w381:cluster{bool[]})  [unwired: 1 in]
      }
      n44 = Bundle("DIOsMod0Name"=w86, "DIOsMod1Name"=w87, "DIOsMod2AName"=w85, "DIOsMod2BName"=w84, "ReglerNameMod0"=w103, "ReglerNameMod1"=w102, "ReglerNameMod2A"=w101, "ReglerNameMod2B"=w100, "LangsameHeizungen"=w174) -> (w236:T18)  [unwired: 1 in]
      n45 = Build Array (concatenate)(w103, w102, w101, w100) -> (w127:string[])
      n46 = Build Array (concatenate)(w196, w195, w194, w193) -> (w247:string[])
      n47 = Build Array (concatenate)(w200, w199, w198, w197) -> (w248:string[])
      n48 = Build Array (concatenate)(w192, w191, w190, w189) -> (w240:dbl[])
      n49 = Build Array (concatenate)(w188, w187, w186, w185) -> (w246:string[])
      n50 = Build Array (concatenate)(w103, w102, w101, w100) -> (→"HorstRegler":string[])
      n51 = Build Array (concatenate)(w49, w48, w47, w46) -> (w45:dbl[][])
      n52 = Array Size(array=w107) -> (size(s)=w106:i32)
      n53 = Build Array(w157, w156, w155, w154) -> (w153:i32[][])
      n54 = Array Size(array=w174) -> (size(s)=w173:i32)
      n55 = Add Array Elements(numeric array=w147) -> (sum=w232:i32)
      n56 = Array Size(array=w144) -> (size(s)=w143:i32)
      n57 = Index Array(array=w113, index=w112) -> (element=w111:T19)
      n58 = Add Array Elements(numeric array=w147) -> (sum=w159:i32)
      n59 = Decrement(x=w169) -> (x-1=w168:i32[])
      n60 = Build Cluster Array(w157, w156, w155, w154) -> (w239:cluster{"DIOsMod2BNr":i32[]}[])
      n61 = Build Array (concatenate)(w180, w179, w178) -> (w118:string[])
      n62 = Index Array(array=w181, index (col)=2 ("Deaktivierter Index (Spalte)")) -> (element=w228:dbl[])  [unwired: 1 in]
      n63 = Index Array(array=w181, index (col)=0 ("Deaktivierter Index (Spalte)")) -> (element=w226:dbl[])  [unwired: 1 in]
      n64 = Index Array(array=w181, index (col)=1 ("Deaktivierter Index (Spalte)")) -> (element=w227:dbl[])  [unwired: 1 in]
      n65 = Concatenate Strings("?SE0,SETP,1700" ("string"), "\r\n") -> (w61:string)
      n66 = Concatenate Strings("?SE0,SETP,1100" ("string"), "\r\n") -> (w68:string)
      n67 = for {
        tunnel: w239 -> [w411] mode=indexing
        tunnel: [w412] -> w238 mode=indexing
        n68 = Unbundle(w411) -> ("DIOsMod2BNr"=w410:i32[])
        n69 = Array Size(array=w410) -> (size(s)=w412:i32)
      }
      n70 = property on="Methode" class="Ring (strict)"("Strings []"=w241) -> ()  [unwired: 2 in, 2 out]
      n71 = Bundle("Modul1/AI sicherer Bereich"=w54, "Modul2/AI sicherer Bereich"=w53, "Modul3/AI sicherer Bereich"=w52, "Traps/Machs sicherer Bereich"=w51, w45, "Metavariablen grüner Bereich"=w44) -> (w50:T20)  [unwired: 1 in]
      n72 = Build Array (concatenate)(w141, w140) -> (w139:dbl[])
      n73 = Array Size(array=w153) -> (size(s)=w152:i32[])
      n74 = Unbundle(w111) -> ("SPMPV"=w110:i32[])  [unwired: 44 out]
      n75 = Open/Create/Replace File(file path (use dialog)=path "c:/fromcriordy.txt" ("Dateipfad (Dialog verwenden)"), operation (0:open)=T14."replace or create" ("Operation (0:Öffnen)")) -> (refnum out=w205:refnum<file>, error out=w206:errorcluster)  [unwired: 4 in, 1 out]
      n76 = Initialize Array(0.0 ("element"), w106) -> (w104:dbl[])
      n77 = Initialize Array(0.0 ("Element"), w159) -> (w158:dbl[])
      n78 = Get Date/Time In Seconds() -> (seconds since 1Jan1904=w98:timestamp)
      n79 = Initialize Array(FALSE, w143) -> (w138:bool[])
      n80 = Multiply(x=w168, y=32) -> (x*y=w171:i32[])
      n81 = Initialize Array(-1.0, w159) -> (w161:dbl[])
      n82 = Array Subset(array=w118, index=32 ("Index"), length=32 ("Länge")) -> (→"AIs2":string[])
      n83 = Array Subset(array=w118, index=0 ("Index"), length=32 ("Länge")) -> (→"AIs1":string[])
      n84 = Array Subset(array=w118, index=64 ("Index"), length=32 ("Länge")) -> (→"AIs3":string[])
      n85 = global write "GVHK1Hz.vi" "Mod1Mod2Mod3/AITrapsMachs1Hz"(w139) -> ()
      n86 = global write "GVMetavariablen.vi" "Metavariablen"(w104) -> ()
      n87 = global write "GVHeizenLH.vi" "Heizen?LH"(w138) -> ()
      n88 = global write "GVZwangs.vi" "ZwangsLangsameHeizungenAn!"(w138) -> ()
      n89 = for {
        tunnel: w152 -> [w391] mode=indexing
        tunnel: [w388] -> w151 mode=indexing
        n90 = Initialize Array(FALSE, w391) -> (w389:bool[])
        n91 = Bundle(w389) -> (w388:cluster{bool[]})  [unwired: 1 in]
      }
      n92 = global write "GVHorstSP.vi" "HorstSP"(w158) -> ()
      n93 = global write "GVZwangs.vi" "ZwangsLangsameHeizungenAn?"(w138) -> ()
      n94 = Add(x=w171, y=w144) -> (x+y=w170:i32[])
      n95 = Close File(refnum=w205, error in=w206) -> (path=w237:path)  [unwired: 1 out]
      n96 = Format Date/Time String(time format string (%c)="%Y-%m-%d--%H-%M" ("Zeitformatierungs-String (%c)"), seconds (now)=w98) -> (date/time string=w76:string)  [unwired: 1 in]
      n97 = String To Byte Array(string=w61) -> (unsigned byte array=w63:u8[])
      n98 = String To Byte Array(string=w68) -> (unsigned byte array=w73:u8[])
      n99 = Index Array(array=w110, index=0) -> (element=w108:i32)
      n100 = global write "GVMWHorst.vi" "MWHorst"(w161) -> ()
      n101 = global write "GVVentilposition.vi" "Ventilposition"(w108) -> ()
      n102 = Build Array (concatenate)(string[] ["Jahr", "Monat", "Tag", "Stunde", "Minute", "Sekunde"] ("Array"), string[] ["Datei Nr.", "Methode Nr.", "Zyklusnr. Mod0", "Zyklusnr. Mod1", "Zyklusnr. Mod2A", "Zyklusnr. Mod2B"], w243, w118, w128, w127, "Probenvolumen1", "Probenvolumen2", "Ventilposition" ("element"), string[] ["CPU Total", "CPU Time critical", "CPU Timed Structures", "CPU High", "CPU Above normal", "CPU Normal", "CPU Background", "CPU Idle", "CPU ISR", "Memory", "SekundenTotalBrutal"]) -> (w245:string[])
      n103 = Build Array (concatenate)(w128, w127) -> (w126:string[])
      n104 = Build Array (concatenate)(w118, w128, w127) -> (w125:string[])
      n105 = Join Numbers(hi=w63, lo=u8 5) -> ((hi.lo)=w60:u16[])
      n106 = Join Numbers(hi=w73, lo=u8 6) -> ((hi.lo)=w71:u16[])
      n107 = Split 1D Array(array=w243, index=2 ("Index")) -> (second subarray=w235:string[])  [unwired: 1 out]
      n108 = call "FPGA-Start-01-17.vi"() -> ("error out"=w59:errorcluster, "FPGA VI Reference Out"=w58:refnum<k20>)  [unwired: 2 in]
      n109 = Concatenate Strings("HK " ("String"), w76) -> (w80:string)
      n110 = Concatenate Strings("ECD1 " ("String"), w76) -> (w78:string)
      n111 = Concatenate Strings("ECD2 " ("String"), w76) -> (w75:string)
      n112 = property on="dargestellte Größe 1" class="Ring (strict)"("Strings []"=w125) -> ()  [unwired: 2 in, 2 out]
      n113 = global write "GVZwangs.vi" "ZwangsHorst!"(w146) -> ()
      n114 = global write "GVZwangs.vi" "ZwangsHorst?"(w145) -> ()
      n115 = xnode "Invoke Method"("FPGA VI Reference In"=w58, "Data"=w60) -> ("FPGA VI Reference Out"=w66:refnum<k20>)  [unwired: 2 in, 2 out]
      n116 = property on="dargestellte Größe 2" class="Ring (strict)"("Strings []"=w125) -> ()  [unwired: 2 in, 2 out]
      n117 = property on="dargestellte Größe 3" class="Ring (strict)"("Strings []"=w126) -> ()  [unwired: 2 in, 2 out]
      n118 = property on="Zeitachse2" class="Ring (strict)"("Strings []"=w235) -> ()  [unwired: 2 in, 2 out]
      n119 = property on="Zeitachse1" class="Ring (strict)"("Strings []"=w235) -> ()  [unwired: 2 in, 2 out]
      n120 = xnode "Invoke Method"("FPGA VI Reference In"=w66, "Data"=w71) -> ("FPGA VI Reference Out"=w57:refnum<k20>)  [unwired: 2 in, 2 out]
      n121 = Build Path(base path=w83, name or relative path=w80) -> (appended path=w91:path)
      n122 = Build Path(base path=w97, name or relative path=w78) -> (appended path=w93:path)
      n123 = Build Path(base path=w96, name or relative path=w75) -> (appended path=w95:path)
      n124 = global write "GVZwangs.vi" "ZwangsDIO!"(w151) -> ()
      n125 = global write "GVZwangs.vi" "ZwangsDIO?"(w151) -> ()
      n126 = Create Folder(path (use dialog)=w91) -> (created path=w90:path)  [unwired: 2 in, 2 out]
      n127 = Create Folder(path (use dialog)=w93) -> (created path=w92:path)  [unwired: 2 in, 2 out]
      n128 = Create Folder(path (use dialog)=w95) -> (created path=w94:path)  [unwired: 2 in, 2 out]
      n129 = call "MPVSenden-01-17.vi"("Ventilposition"=0, "FPGA VI Reference In"=w57) -> ("FPGA VI Reference Out"=w55:refnum<k20>)  [unwired: 1 in, 2 out]
      n130 = case shown="True" w114 {
        tunnel: [w402 w407] -> w219
        tunnel: [w402 w406] -> w218
        tunnel: w90 -> [_ w405]
        tunnel: w177 -> [_ w404]
        tunnel: w112 -> [_ w403]
        frame False {
          w402 = refnum<k34> refnum ("tdms1")
        }
        frame True {
          n131 = call "TDMS0.vi"("Startmethode"=w403, "Dateiname"=w404, "Dateiordner"=w405) -> ("tdms1"=w406:refnum<k34>, "tdms0"=w407:refnum<k34>)
          n132 = global write "GVaktuelleTDMS.vi" "aktuelleTDMS-DateiHK"(w407) -> ()
        }
      }
      n133 = case shown="True" w114 {
        tunnel: [w392 w401] -> w217
        tunnel: [w392 w400] -> w216
        tunnel: [w392 w399] -> w215
        tunnel: [w392 w398] -> w214
        tunnel: w92 -> [_ w397]
        tunnel: w176 -> [_ w396]
        tunnel: w94 -> [_ w395]
        tunnel: w175 -> [_ w394]
        tunnel: w112 -> [_ w393]
        frame False {
          w392 = refnum<k34> refnum ("tdms0")
        }
        frame True {
          n134 = call "TDMS0.vi"("Startmethode"=w393, "Dateiname"=w396, "Dateiordner"=w397) -> ("tdms1"=w400:refnum<k34>, "tdms0"=w401:refnum<k34>)
          n135 = call "TDMS0.vi"("Startmethode"=w393, "Dateiname"=w394, "Dateiordner"=w395) -> ("tdms1"=w398:refnum<k34>, "tdms0"=w399:refnum<k34>)
          n136 = global write "GVaktuelleTDMS.vi" "aktuelleTDMS-DateiECD1"(w401) -> ()
          n137 = global write "GVaktuelleTDMS.vi" "aktuelleTDMS-DateiECD2"(w399) -> ()
        }
      }
      n138 = Open/Create/Replace File(file path (use dialog)=path "c:/fromcriocmd.txt" ("Pfad MS-Datei CRIO"), operation (0:open)=T14."replace or create" ("Operation (0:Öffnen)")) -> (refnum out=w211:refnum<file>, error out=w210:errorcluster)  [unwired: 4 in, 1 out]
      n139 = Write to Text File(file (use dialog)=w211, text="time=yyyymmddhhmmss\ncycle=005\ninfo=1234567890123456789012345678901234567890123456789012345678901234567890123456789012345678901234567890\nlength=100\ncmd=cycle" ("Text0 MS-Datei"), error in=w210) -> (refnum out=w208:refnum<file>, error out=w207:errorcluster)  [unwired: 1 in, 1 out]
      n140 = Bundle("created path"=w90, "created path"=w92, "created path"=w94, "Dateiname Housekeeping"=w177, "DateinameECD1"=w176, "DateinameECD2"=w175, "tdms0"=w219, "tdms1"=w218, "tdms0"=w217, "tdms1"=w216, "tdms0"=w215, "tdms1"=w214) -> (w220:T21)  [unwired: 1 in]
      n141 = call "AIKoeffSortieren.vi"("Modul3/AI koeff"=w182, "Modul2/AI koeff"=w183, "Modul1/AI koeff"=w184) -> ("P0"=w223:dbl[], "P1"=w224:dbl[], "P2"=w225:dbl[])
      n142 = Close File(refnum=w208, error in=w207) -> (path=w202:path)  [unwired: 1 out]
      "schnelle Heizungen" <- string[] ["Trap1 [°C]", "Trap2 [°C]", "PreCol1 [°C]", "PreCol2 [°C]", "MainCol1 [°C]", "MainCol2 [°C]"]
    }
    frame #1 {
      w421 = dbl[] [-1.0]
      w492 = 0
      w467 = 0 ("Zyklusnummer1")
      n143 = flat-sequence {
        frame #0 {
          n144 = global write "Emulate Licor output GV.vi" "Emulator an?"(FALSE ("Emulator an?")) -> ()
        }
        frame #1 {
          n145 = control-ref of="GUI_Cluster_sdv"() -> (w520:refnum<vi>)
          n146 = control-ref of="GUI_Cluster_Graph"() -> (w522:refnum<vi>)
          n147 = control-ref of="GUI_Cluster_Parameter"() -> (w521:refnum<vi>)
          n148 = call "licore (main).vi"("GUI_Cluster_Graph (extern)"=w522, "GUI_Cluster_Parameter (extern)"=w521, "GUI_Cluster_sdv (extern)"=w520) -> ()  [unwired: 13 in]
        }
      }
      n149 = while {
        stop <- w1336 stop-if-true
        w1330 = 10.0
        n150 = call "Warten2"("Count(mSec)"=u32 1000) -> ()  [unwired: 1 out]
        n151 = global read "gvbooleschRT.vi" "global stop RT"() -> (w1336:bool)
        n152 = global read "GVTrapsMachs.vi" "Traps/Machs"() -> (w1326:dbl[])
        n153 = global read "GVAIs.vi" "AIs"() -> (w1327:dbl[])
        n154 = for {
          N: 9 -> [_]
          shift-right: [w1339] -> w1333
          shift-left: w1327 -> [w1340]
          shift-right: [w1337] -> w1331
          shift-left: w1326 -> [w1338]
          n155 = flat-sequence {
            tunnel: w1340 -> [w1347]
            tunnel: [w1346] -> w1339
            tunnel: w1338 -> [w1345]
            tunnel: [w1344] -> w1337
            frame #0 {
              n156 = call "Warten28"("Count(mSec)"=u32 100) -> ()  [unwired: 1 out]
            }
            frame #1 {
              n157 = global read "GVAIs.vi" "AIs"() -> (w1343:dbl[])
              n158 = Add(x=w1347, y=w1343) -> (x+y=w1346:dbl[])
              n159 = global read "GVTrapsMachs.vi" "Traps/Machs"() -> (w1342:dbl[])
              n160 = Add(x=w1342, y=w1345) -> (x+y=w1344:dbl[])
            }
          }
        }
        n161 = Divide(x=w1333, y=w1330) -> (x/y=w1332:dbl[])
        n162 = Divide(x=w1331, y=w1330) -> (x/y=w1329:dbl[])
        n163 = Build Array (concatenate)(w1332, w1329) -> (w1328:dbl[])
        n164 = global write "GVHK1Hz.vi" "Mod1Mod2Mod3/AITrapsMachs1Hz"(w1328) -> ()
      }
      n165 = while {
        shift-right: ["Methode"] -> _
        shift-left: w518 -> [w1350]
        stop <- w1352 stop-if-true
        n166 = call "Bis zum nächsten Vielfachen warten7"("Count(mSec)"=u32 1000) -> ()  [unwired: 1 out]
        n167 = Not Equal?(x=w1350, y="Methode") -> (x != y?=w1348:bool)
        n168 = global read "gvbooleschRT.vi" "global stop RT"() -> (w1352:bool)
        n169 = global write "GVMethodenwechsel.vi" "Methodenwechsel?"(w1348) -> ()
      }
      n170 = Add Array Elements(numeric array=w441) -> (sum=w440:i32)
      n171 = Array Size(array=w449) -> (size(s)=w470:i32)
      n172 = Unbundle(w466) -> ("created path"=w465:path, "created path"=w463:path, "created path"=w462:path, "Dateiname Housekeeping"=w464:string, "DateinameECD1"=w461:string, "DateinameECD2"=w460:string, "tdms0"=w459:refnum<k34>, "tdms1"=w458:refnum<k34>, "tdms0"=w457:refnum<k34>, "tdms1"=w456:refnum<k34>, "tdms0"=w455:refnum<k34>, "tdms1"=w454:refnum<k34>)
      n173 = Index Array(array=w442, index #1=0 ("Index"), index #2=1 ("Index"), index #3=2 ("Index"), index #4=3 ("Index")) -> (element #1=w481:i32, element #2=w480:i32, element #3=w483:i32, element #4=w482:i32)
      n174 = call <vilib>:"Space Constant.vi"() -> ("String"=w427:string)
      n175 = case shown="True" TRUE ("ECDSpeichern") {
        frame False {
        }
        frame True {
          w828 = dbl[] []
          n176 = global read "GVaktuelleTDMS.vi" "aktuelleTDMS-DateiECD1"() -> (w829:refnum<k34>)
          n177 = while {
            shift-right: [w841] -> _
            shift-left: w828 -> [w845]
            shift-right: [w834] -> _
            shift-left: w828 -> [w838]
            shift-right: [w840] -> _
            shift-left: w829 -> [w843]
            tunnel: w828 -> [w837]
            shift-right: [w831] -> _
            shift-left: errorcluster {"status"=FALSE, "code"=0, "source"=""} ("error IO") -> [w830]
            stop <- w850 stop-if-true
            n178 = call "Bis zum nächsten Vielfachen warten3"("Count(mSec)"=u32 500) -> ()  [unwired: 1 out]
            n179 = global read "GVECDs.vi" "ECD1MW"() -> (w844:dbl[])
            n180 = global read "GVECDs.vi" "ECD2MW"() -> (w835:dbl[])
            n181 = global read "gvbooleschRT.vi" "global stop RT"() -> (w850:bool)
            n182 = Build Array (concatenate)(w845, w844) -> (w842:dbl[])
            n183 = Build Array (concatenate)(w838, w835) -> (w839:dbl[])
            n184 = global read "GVaktuelleTDMS.vi" "aktuelleTDMS-DateiECD1"() -> (w840:refnum<k34>)
            n185 = global read "GVaktuelleTDMS.vi" "aktuelleTDMS-DateiECD2"() -> (w848:refnum<k34>)
            n186 = Equal?(x=w843, y=w840) -> (x = y?=w836:bool)
            n187 = TDMS Write(0:w840, 7:"ECD1", 9:w844, 11:w830) -> (15:w833:errorcluster)  [unwired: 2 in, 3 out]
            n188 = TDMS Write(0:w848, 7:"ECD2", 9:w835, 11:w830) -> (15:w832:errorcluster)  [unwired: 2 in, 3 out]
            n189 = Select(t=w842, s=w836, f=w837) -> (s? t:f=w841:dbl[])
            n190 = Select(t=w839, s=w836, f=w837) -> (s? t:f=w834:dbl[])
            n191 = global write "GVChroms.vi" "ECD1Chrom"(w841) -> ()
            n192 = global write "GVChroms.vi" "ECD2Chrom"(w834) -> ()
            n193 = Merge Errors(w833, w832) -> (w831:errorcluster)
            "TDMSwriteECD" <- w831
          }
        }
      }
      n194 = while {
        shift-right: [w525] -> _
        shift-left: w421 -> [w527]
        shift-right: [w524] -> _
        shift-left: w421 -> [w526]
        stop <- w529 stop-if-true
        n195 = call "Bis zum nächsten Vielfachen warten"("Count(mSec)"=u32 100) -> ()  [unwired: 1 out]
        n196 = case shown="True" "An/Aus" {
          tunnel: w527 -> [w531 w547]
          tunnel: w526 -> [w530 w546]
          tunnel: [w531 w540] -> w525
          tunnel: [w530 w539] -> w524
          frame False {
          }
          frame True {
            w543 = dbl[] [] ("t")
            n197 = global read "GVMWHorst.vi" "MWHorst"() -> (w536:dbl[])
            n198 = global read "GVTrapsMachs.vi" "Traps/Machs"() -> (w537:dbl[])
            n199 = Build Array (concatenate)(w537, w536) -> (w535:dbl[])
            n200 = Index Array(array=w535, index="dargestellte Größe 3") -> (element=w548:dbl)
            n201 = Build Array (concatenate)(w547, w548) -> (w541:dbl[])
            n202 = Select(t=w543, s="TafelWischen!", f=w541) -> (s? t:f=w540:dbl[])
            n203 = global read "GVZeitenZyklen.vi" "Big Ben, Methodenzeit, Zykluszeit0, Zykluszeit1, Zykluszeit2A, Zykluszeit2B"() -> (w534:dbl[])
            n204 = Index Array(array=w534, index=1 ("Index")) -> (element=w532:dbl)
            n205 = Build Array (concatenate)(w546, w532) -> (w542:dbl[])
            n206 = Select(t=w543, s="TafelWischen!", f=w542) -> (s? t:f=w539:dbl[])
            n207 = Bundle(w542, w541) -> (→"schnelleAnzeige":cluster{dbl[], dbl[]})  [unwired: 1 in]
          }
        }
        n208 = global read "gvbooleschRT.vi" "global stop RT"() -> (w529:bool)
      }
      n209 = while {
        tunnel: w445 -> [w893]
        tunnel: w514 -> [w892]
        tunnel: w513 -> [w891]
        tunnel: w512 -> [w890]
        shift-right: [w889] -> _
        shift-left: errorcluster {"status"=FALSE, "code"=0, "source"=""} ("error out") -> [w888]
        stop <- w894 stop-if-true
        n210 = call "AIsFIFORT-01-17.vi"("FPGA VI Reference In"=w893, "P2"=w892, "P1"=w891, "P0"=w890, "error in"=w888) -> ("error out"=w889:errorcluster)
        "AIsFIFOread" <- w889
        n211 = global read "gvbooleschRT.vi" "global stop RT"() -> (w894:bool)
      }
      n212 = while {
        tunnel: w445 -> [w895]
        tunnel: w420 -> [w900]
        tunnel: w419 -> [w899]
        tunnel: w418 -> [w898]
        shift-right: [w897] -> _
        shift-left: errorcluster {"status"=FALSE, "code"=0, "source"=""} ("error out") -> [w896]
        stop <- w902 stop-if-true
        n213 = call "TrapsMachMitteln-01-17.vi"("FPGA VI Reference In"=w895, "Traps/MachKoeff2"=w900, "Traps/MachKoeff1"=w899, "Traps/MachKoeff0"=w898, "error in"=w896) -> ("error out"=w897:errorcluster)
        "MWTrapsMachs" <- w897
        n214 = call "Bis zum nächsten Vielfachen warten16"("Count(mSec)"=u32 100) -> ()  [unwired: 1 out]
        n215 = global read "gvbooleschRT.vi" "global stop RT"() -> (w902:bool)
      }
      n216 = case shown="True" TRUE ("HKSpeichern") {
        tunnel: w516 -> [_ w881]
        frame False {
        }
        frame True {
          n217 = while {
            tunnel: w881 -> [w885]
            shift-right: [w883] -> _
            shift-left: errorcluster {"status"=FALSE, "code"=0, "source"=""} ("error out") -> [w882]
            stop <- w887 stop-if-true
            n218 = call "Bis zum nächsten Vielfachen warten2"("Count(mSec)"=u32 1000) -> ()  [unwired: 1 out]
            n219 = local read "Methode"() -> (w884:i32)
            n220 = global read "gvbooleschRT.vi" "global stop RT"() -> (w887:bool)
            n221 = call "HKinTDMS-01-16.vi"("Methode"=w884, "error in (no error)"=w882, "Kanäle"=w885) -> ("error out"=w883:errorcluster)
            "TDMSwriteHK" <- w883
          }
        }
      }
      n222 = for {
        N: 1 -> [_]
        tunnel: w445 -> [w903]
        tunnel: [w903] -> w472
        n223 = call "Warten8"("Count(mSec)"=u32 100) -> ()  [unwired: 1 out]
      }
      n224 = Build Array(w427) -> (w426:string[])
      n225 = Initialize Array(-1 ("Element"), 4 ("Dimension")) -> (w443:i32[])
      n226 = global read "GVVentilposition.vi" "Ventilposition"() -> (w451:i32)
      n227 = case shown="True" TRUE {
        tunnel: w467 -> [_ w860]
        tunnel: w465 -> [_ w859]
        tunnel: w464 -> [_ w858]
        tunnel: w459 -> [_ w857]
        tunnel: w458 -> [_ w856]
        frame False {
        }
        frame True {
          w851 = errorcluster {"status"=FALSE, "code"=0, "source"=""} ("error out TDMSopen")
          n228 = while {
            shift-right: [w865] -> w855
            shift-left: w857 -> [w867]
            shift-right: [w876] -> w854
            shift-left: w856 -> [w869]
            shift-right: [w871] -> _
            shift-left: w860 -> [w877]
            tunnel: w858 -> [w873]
            tunnel: w859 -> [w874]
            shift-right: [w864] -> w853
            shift-left: w851 -> [w862]
            shift-right: [w863] -> w852
            shift-left: w851 -> [w861]
            stop <- w879 stop-if-true
            n229 = call "Bis zum nächsten Vielfachen warten5"("Count(mSec)"=u32 500) -> ()  [unwired: 1 out]
            n230 = local read "Methode"() -> (w875:i32)
            n231 = global read "gvbooleschRT.vi" "global stop RT"() -> (w879:bool)
            n232 = global read "GVZeitenZyklen.vi" "ZyklusNummernGesamt"() -> (w866:i32[])
            n233 = Index Array(array=w866, index=1 ("Index")) -> (element=w871:i32)
            n234 = Greater?(x=w871, y=w877) -> (0:w870:bool)
            n235 = Select(t=w869, s=w870, f=w867) -> (s? t:f=w868:refnum<k34>)
            n236 = call "AktuelleTDMS.vi"("AktuelleTDMS"=w867, "error in TDMSopen"=w862, "Dateiordner"=w874, "NächsteTDMS"=w869, "NeuerZyklus?"=w870, "Methodennummer"=w875, "Zyklnumges"=w871, "error in TDMSclose"=w861, "Dateiname"=w873) -> ("AktuelleTDMS"=w865:refnum<k34>, "error out TDMSopen"=w864:errorcluster, "error out TDMSclose"=w863:errorcluster, "NächsteTDMS"=w876:refnum<k34>)  [unwired: 3 in]
            "TDMSopenHK" <- w864
            "TDMScloseHK" <- w863
            n237 = global write "GVaktuelleTDMS.vi" "aktuelleTDMS-DateiHK"(w868) -> ()
          }
          n238 = TDMS Close(8:w853, 11:w855) -> ()  [unwired: 2 out]
          n239 = TDMS Close(8:w852, 11:w854) -> ()  [unwired: 2 out]
        }
      }
      n240 = case shown="True" TRUE {
        tunnel: w467 -> [_ w788]
        tunnel: w463 -> [_ w787]
        tunnel: w462 -> [_ w786]
        tunnel: w461 -> [_ w785]
        tunnel: w460 -> [_ w784]
        tunnel: w457 -> [_ w783]
        tunnel: w456 -> [_ w782]
        tunnel: w455 -> [_ w781]
        tunnel: w454 -> [_ w780]
        frame False {
        }
        frame True {
          w773 = errorcluster {"status"=FALSE, "code"=0, "source"=""} ("error out TDMSopen")
          n241 = while {
            shift-right: [w812] -> w779
            shift-left: w783 -> [w814]
            shift-right: [w822] -> w778
            shift-left: w782 -> [w816]
            shift-right: [w820] -> _
            shift-left: w788 -> [w823]
            tunnel: w787 -> [w819]
            tunnel: w785 -> [w818]
            shift-right: [w811] -> w774
            shift-left: w773 -> [w809]
            shift-right: [w810] -> w775
            shift-left: w773 -> [w808]
            stop <- w825 stop-if-true
            n242 = call "Bis zum nächsten Vielfachen warten4"("Count(mSec)"=u32 500) -> ()  [unwired: 1 out]
            n243 = local read "Methode"() -> (w821:i32)
            n244 = global read "gvbooleschRT.vi" "global stop RT"() -> (w825:bool)
            n245 = global read "GVZeitenZyklen.vi" "ZyklusNummernGesamt"() -> (w813:i32[])
            n246 = Index Array(array=w813, index=2 ("Index")) -> (element=w820:i32)
            n247 = Greater?(x=w820, y=w823) -> (0:w817:bool)
            n248 = Select(t=w816, s=w817, f=w814) -> (s? t:f=w815:refnum<k34>)
            n249 = call "AktuelleTDMS.vi"("AktuelleTDMS"=w814, "error in TDMSopen"=w809, "Dateiordner"=w819, "NächsteTDMS"=w816, "NeuerZyklus?"=w817, "Methodennummer"=w821, "Zyklnumges"=w820, "error in TDMSclose"=w808, "Dateiname"=w818) -> ("AktuelleTDMS"=w812:refnum<k34>, "error out TDMSopen"=w811:errorcluster, "error out TDMSclose"=w810:errorcluster, "NächsteTDMS"=w822:refnum<k34>)  [unwired: 3 in]
            "TDMSopenECD1" <- w811
            "TDMScloseECD1" <- w810
            n250 = global write "GVaktuelleTDMS.vi" "aktuelleTDMS-DateiECD1"(w815) -> ()
          }
          n251 = while {
            shift-right: [w802] -> w777
            shift-left: w781 -> [w794]
            shift-right: [w803] -> w776
            shift-left: w780 -> [w796]
            shift-right: [w800] -> _
            shift-left: w788 -> [w804]
            tunnel: w786 -> [w799]
            tunnel: w784 -> [w798]
            shift-right: [w792] -> _
            shift-left: w773 -> [w790]
            shift-right: [w791] -> _
            shift-left: w773 -> [w789]
            stop <- w806 stop-if-true
            n252 = call "Bis zum nächsten Vielfachen warten6"("Count(mSec)"=u32 500) -> ()  [unwired: 1 out]
            n253 = local read "Methode"() -> (w801:i32)
            n254 = global read "gvbooleschRT.vi" "global stop RT"() -> (w806:bool)
            n255 = global read "GVZeitenZyklen.vi" "ZyklusNummernGesamt"() -> (w793:i32[])
            n256 = Index Array(array=w793, index=3 ("Index")) -> (element=w800:i32)
            n257 = Greater?(x=w800, y=w804) -> (0:w797:bool)
            n258 = Select(t=w796, s=w797, f=w794) -> (s? t:f=w795:refnum<k34>)
            n259 = call "AktuelleTDMS.vi"("AktuelleTDMS"=w794, "error in TDMSopen"=w790, "Dateiordner"=w799, "NächsteTDMS"=w796, "NeuerZyklus?"=w797, "Methodennummer"=w801, "Zyklnumges"=w800, "error in TDMSclose"=w789, "Dateiname"=w798) -> ("AktuelleTDMS"=w802:refnum<k34>, "error out TDMSopen"=w792:errorcluster, "error out TDMSclose"=w791:errorcluster, "NächsteTDMS"=w803:refnum<k34>)  [unwired: 3 in]
            "TDMSopenECD2" <- w792
            "TDMScloseECD2" <- w791
            n260 = global write "GVaktuelleTDMS.vi" "aktuelleTDMS-DateiECD2"(w795) -> ()
          }
          n261 = TDMS Close(8:w774, 11:w779) -> ()  [unwired: 2 out]
          n262 = TDMS Close(8:w775, 11:w778) -> ()  [unwired: 2 out]
          n263 = TDMS Close(11:w777) -> ()  [unwired: 1 in, 2 out]
          n264 = TDMS Close(11:w776) -> ()  [unwired: 1 in, 2 out]
        }
      }
      n265 = Add(x=w483, y=w482) -> (x+y=w479:i32)
      n266 = Bundle(w426, w426, w426) -> (w490:cluster{string[], string[], string[]})  [unwired: 1 in]
      n267 = Index Array(array=w436, index=w434) -> (element=w435:T19)
      n268 = Initialize Array(cluster{"output high":dbl, "output low":dbl} {"output high"=99999.0, "output low"=0.0} ("output range"), w470) -> (w450:cluster{"output high":dbl, "output low":dbl}[])
      n269 = Concatenate Strings("?SE0,GDATA" ("Schreibpuffer"), "\r") -> (w422:string)
      n270 = Build Array(w481, w480, w479) -> (w478:i32[])
      n271 = while {
        tunnel: w517 -> [w1030]
        shift-right: [w1029] -> _
        shift-left: w436 -> [w1011]
        tunnel: w450 -> [w1028]
        tunnel: w449 -> [w1027]
        tunnel: w445 -> [w1026]
        tunnel: w448 -> [w1025]
        tunnel: w447 -> [w1024]
        shift-right: [w1018] -> _
        shift-left: 0 -> [w1023]
        tunnel: w445 -> [w1022]
        tunnel: w444 -> [w1021]
        shift-right: [w1017] -> _
        shift-left: w443 -> [w1020]
        tunnel: w442 -> [w1012]
        tunnel: w441 -> [w1013]
        tunnel: w440 -> [w1014]
        tunnel: w439 -> [w1015]
        tunnel: w438 -> [w1016]
        tunnel: w437 -> [w1019]
        shift-right: [w934] -> _
        shift-left: w435 -> [w933]
        tunnel: w420 -> [w912]
        tunnel: w419 -> [w916]
        tunnel: w418 -> [w922]
        tunnel: w413 -> [w905]
        i -> [w937]
        stop <- w1031 stop-if-true
        w923 = 0  # ZeileMainMach2
        w924 = 0  # ZeileMainMach1
        w979 = FALSE
        w978 = 0.0
        w980 = 0  # ZeilennummerMPV
        w984 = cluster{dbl[], dbl[]} {[], []}
        w993 = dbl[] []
        w997 = 0  # ZeilePreMach2
        w998 = 0  # ZeilePreMach1
        w999 = 0  # ZeileFPGAFixp
        w1000 = 0  # ZeileFPGAPID
        w1001 = 0  # ZeileFPGABoolesch
        w1002 = i32[] [0, 0, 0, 0]  # ZeilennummernHorst
        w1003 = i32[] [0, 0, 0, 0]  # ZeilennummernDIOs
        n272 = Unbundle(w933) -> ("Zykluslängen [s]"=w977:dbl[], "ZeitpktDIOsMod0"=w976:dbl[], "ZeitpktDIOsMod1"=w975:dbl[], "ZeitpktDIOsMod2A"=w974:dbl[], "ZeitpktDIOsMod2B"=w973:dbl[], "DIOsSPMod0"=w972:bool[][], "DIOsSPMod1"=w971:bool[][], "DIOsSPMod2A"=w970:bool[][], "DIOsSPMod2B"=w969:bool[][], "Mod0HorstZeitpkt"=w968:dbl[], "Mod1HorstZeitpkt"=w967:dbl[], "Mod2AHorstZeitpkt"=w966:dbl[], "Mod2BHorstZeitpkt"=w965:dbl[], "HorstSPMod0"=w964:dbl[][], "HorstSPMod1"=w963:dbl[][], "HorstSPMod2A"=w962:dbl[][], "HorstSPMod2B"=w961:dbl[][], "LHSetpoints"=w960:dbl[], "LHHeizen?"=w959:bool[], "ZPktFPGABoolesch"=w958:dbl[], "FPGABoolesch"=w957:bool[][], "ZeitpktFPGAPID"=w956:dbl[], "FPGAPID"=w955:T22, "ZeitpktFPGAFixp"=w954:dbl[], "SHSetpoints"=w953:dbl[][], "t_PreMach1"=w952:dbl[], "T_PreMach1"=w951:dbl[], "t_PreMach2"=w950:dbl[], "T_PreMach2"=w949:dbl[], "PIDs für \"träge\" Heizungen"=w948:T23, "Zwangsbedingungen"=w947:dbl[][], "Dateien fürs MS schicken?"=w946:bool, "ZeitpunkteMPV"=w945:dbl[], "SPMPV"=w944:i32[], "ZeitpktMS-1"=w943:dbl, "ZeitpktMS-2"=w942:dbl, "Int.Start1"=w941:dbl, "Int.Stop1"=w940:dbl, "Int.Start2"=w939:dbl, "Int.Stop2"=w938:dbl, "t_MainMach1"=w932:dbl[], "T_MainMach1"=w931:dbl[], "t_MainMach2"=w930:dbl[], "T_MainMach2"=w929:dbl[])  [unwired: 1 out]
        n273 = Add(x=w1020, y=1) -> (x+y=w988:i32[])
        n274 = Array Subset(array=w922, index=2 ("Index"), length=4 ("Länge")) -> (w919:dbl[])
        n275 = Array Subset(array=w912, index=2 ("Index"), length=4 ("Länge")) -> (w911:dbl[])
        n276 = Array Subset(array=w916, index=2 ("Index"), length=4 ("Länge")) -> (w915:dbl[])
        n277 = local read "Methode"() -> (w936:i32)
        n278 = while {
          tunnel: w1013 -> [w1104]
          tunnel: w1016 -> [w1102]
          tunnel: w1015 -> [w1101]
          tunnel: w1012 -> [w1103]
          tunnel: w1014 -> [w1100]
          tunnel: w947 -> [w1092]
          stop <- w1094 stop-if-true
          n279 = call "Bis zum nächsten Vielfachen warten10"("Count(mSec)"=u32 1000) -> ()  [unwired: 1 out]
          n280 = local read "Methode"() -> (w1099:i32)
          n281 = global read "GVMethodenwechsel.vi" "Methodenwechsel?"() -> (w1096:bool)
          n282 = global read "gvbooleschRT.vi" "global stop RT"() -> (w1097:bool)
          n283 = case shown="True" "global stop RT" {
            frame False {
            }
            frame True {
              n284 = global write "gvbooleschRT.vi" "global stop RT"(TRUE ("global stop RT")) -> ()
            }
          }
          n285 = call "ZwangsbedingungenGV.vi"("AnzahlHorst"=w1102, "AnzahlHorst/Modul"=w1103, "AnzahlLH"=w1101, "AnzahlDIOs/Modul"=w1104, "AnzahlDIOs"=w1100, "Zwangsbedingungen"=w1092, "Methodennummer"=w1099) -> ("Methodennummer"=w1098:i32)  [unwired: 4 in]
          n286 = local write "Methode"(w1098) -> ()
          n287 = local read "veränderte Methode benutzen"() -> (w1095:bool)
          n288 = Compound Arithmetic op=OR(w1097, w1096, w1095) -> (w1094:bool)
        }
        n289 = Build Cluster Array(w972, w971, w970, w969) -> (w1007:cluster{"DIOsSPMod2B":bool[][]}[])
        n290 = Build Cluster Array(w964, w963, w962, w961) -> (w1005:cluster{"HorstSPMod2B":dbl[][]}[])
        n291 = Build Cluster Array(w976, w975, w974, w973) -> (w1008:cluster{"ZeitpktDIOsMod2B":dbl[]}[])
        n292 = Build Cluster Array(w968, w967, w966, w965) -> (w1006:cluster{"Mod2BHorstZeitpkt":dbl[]}[])
        n293 = Bundle(w919, w915, w911) -> (w910:cluster{dbl[], dbl[], dbl[]})  [unwired: 1 in]
        n294 = Equal?(x=w937, y=0) -> (x = y?=w1009:bool)
        n295 = global read "GVZeitenZyklen.vi" "ZyklusNummern"() -> (w987:i32[])
        n296 = global read "GVZwangs.vi" "ZwangsHorst?"() -> (w992:cluster{bool[]}[])
        n297 = global read "gvbooleschRT.vi" "global stop RT"() -> (w1031:bool)
        n298 = global read "GVZwangsMPV.vi" "ZwangsMPV?"() -> (w908:bool)
        n299 = global read "GVZwangs.vi" "ZwangsDIO?"() -> (w991:cluster{bool[]}[])
        n300 = global read "GVaktuelleTDMS.vi" "aktuelleTDMS-DateiECD1"() -> (w986:refnum<k34>)
        n301 = while {
          tunnel: w1027 -> [w1083]
          tunnel: w1028 -> [w1085]
          tunnel: w1026 -> [w1080]
          tunnel: w960 -> [w1084]
          tunnel: w948 -> [w1086]
          shift-right: [w1082] -> _
          shift-left: errorcluster {"status"=FALSE, "code"=0, "source"=""} ("error out") -> [w1081]
          stop <- w1087 stop-if-true
          n302 = call "LH-01-17.vi"("FPGA VI Reference In"=w1080, "OutputRange"=w1085, "LHSetpoints"=w1084, "AIsLH"=w1083, "error in"=w1081, "PIDs für \"träge\" Heizungen"=w1086) -> ("error out"=w1082:errorcluster)  [unwired: 1 in]
          "LH" <- w1082
          n303 = call "Bis zum nächsten Vielfachen warten12"("Count(mSec)"=u32 100) -> ()  [unwired: 1 out]
          n304 = global read "GVMethodenwechsel.vi" "Methodenwechsel?"() -> (w1089:bool)
          n305 = global read "gvbooleschRT.vi" "global stop RT"() -> (w1090:bool)
          n306 = local read "veränderte Methode benutzen"() -> (w1088:bool)
          n307 = Compound Arithmetic op=OR(w1090, w1089, w1088) -> (w1087:bool)
        }
        n308 = while {
          shift-right: [w1044] -> _
          shift-left: w979 -> [w1048]
          shift-right: [w1043] -> _
          shift-left: w978 -> [w1047]
          shift-right: [w1042] -> _
          shift-left: w979 -> [w1046]
          shift-right: [w1041] -> _
          shift-left: w978 -> [w1045]
          tunnel: w1019 -> [w1040]
          tunnel: w941 -> [w1035]
          tunnel: w940 -> [w1034]
          tunnel: w939 -> [w1033]
          tunnel: w938 -> [w1032]
          stop <- w1037 stop-if-true
          n309 = call "Integrieren.vi"("Integrieren1"=w1048, "Integral1"=w1047, "Integrieren2"=w1046, "Integral2"=w1045, "Int.Start1"=w1035, "Int.Stop1"=w1034, "Int.Start2"=w1033, "HorstProbenflußNr."=w1040, "Int.Stop2"=w1032) -> ("Integrieren1"=w1044:bool, "Integral1"=w1043:dbl, "Integrieren2"=w1042:bool, "Integral2"=w1041:dbl)  [unwired: 7 in]
          n310 = call "Bis zum nächsten Vielfachen warten9"("Count(mSec)"=u32 100) -> ()  [unwired: 1 out]
          n311 = global read "GVMethodenwechsel.vi" "Methodenwechsel?"() -> (w1038:bool)
          n312 = global read "gvbooleschRT.vi" "global stop RT"() -> (w1039:bool)
          n313 = local read "veränderte Methode benutzen"() -> (w1036:bool)
          n314 = Compound Arithmetic op=OR(w1039, w1038, w1036) -> (w1037:bool)
        }
        n315 = while "Zeit" {
          tunnel: w1009 -> [w1287]
          tunnel: w977 -> [w1285]
          tunnel: w988 -> [w1280]
          tunnel: [w1279] -> w1017
          shift-right: [w1276] -> _
          shift-left: 0.0 -> [w1277]
          i -> [w1289]
          stop <- w1282 stop-if-true
          n316 = Equal?(x=w1289, y=0) -> (x = y?=w1278:bool)
          n317 = call "Bis zum nächsten Vielfachen warten15"("Count(mSec)"=u32 50) -> ()  [unwired: 1 out]
          n318 = call "BigBen-01-16.vi"("MethodenStartzeit"=w1277, "Methodenstart?"=w1278, "Programmstart?"=w1287, "Zykluslängen [s]"=w1285, "MethodenStartZyklusNummern"=w1280) -> ("MethodenStartzeit"=w1276:dbl, "ZyklusNummernGesamt"=w1279:i32[])  [unwired: 2 in]
          n319 = global read "GVMethodenwechsel.vi" "Methodenwechsel?"() -> (w1281:bool)
          n320 = global read "gvbooleschRT.vi" "global stop RT"() -> (w1286:bool)
          n321 = Or(x=w1281, y=w1286) -> (x .or. y?=w1283:bool)
          n322 = local read "veränderte Methode benutzen"() -> (w1284:bool)
          n323 = Or(x=w1284, y=w1283) -> (x .or. y?=w1282:bool)
        }
        n324 = Bundle(w1008, w1007, w1006, w1005, "LHHeizen?"=w959, "ZPktFPGABoolesch"=w958, "FPGABoolesch"=w957, "ZeitpktFPGAPID"=w956, "FPGAPID"=w955, "ZeitpktFPGAFixp"=w954, "SHSetpoints"=w953, "t_PreMach1"=w952, "T_PreMach1"=w951, "t_PreMach2"=w950, "T_PreMach2"=w949, "ZeitpunkteMPV"=w945, "SPMPV"=w944, "t_MainMach1"=w932, "T_MainMach1"=w931, "t_MainMach2"=w930, "T_MainMach2"=w929) -> (w1004:T24)  [unwired: 1 in]
        n325 = Index Array(array=w1011, index=w936) -> (element=w935:T19)
        n326 = global read "GVZwangs.vi" "ZwangsFPGABoolesch?"() -> (w990:bool[])
        n327 = while {
          tunnel: w1030 -> [w1302]
          shift-right: [w1293] -> _
          shift-left: w935 -> [w1301]
          tunnel: w936 -> [w1299]
          shift-right: [w1291] -> w1029
          shift-left: w1011 -> [w1300]
          tunnel: [w1292] -> w934
          stop <- w1295 stop-if-true
          n328 = call "Bis zum nächsten Vielfachen warten8"("Count(mSec)"=u32 500) -> ()  [unwired: 1 out]
          n329 = global read "GVMethodenwechsel.vi" "Methodenwechsel?"() -> (w1297:bool)
          n330 = global read "gvbooleschRT.vi" "global stop RT"() -> (w1296:bool)
          n331 = case shown="True" "Methode verändern" {
            tunnel: w1302 -> [_ w1324]
            tunnel: w1301 -> [w1321 w1323]
            tunnel: [w1321 w1322] -> w1293
            frame False {
            }
            frame True {
              n332 = call "methodeändern-11-15.vi"("Methode"=w1323, "Namen"=w1324) -> ("Methode"=w1322:T25)  [unwired: 1 in]
              n333 = property on="Methode verändern" class="Bool (strict)"("Value"=FALSE ("Methode verändern")) -> ()  [unwired: 2 in, 2 out]
            }
          }
          n334 = Compound Arithmetic op=OR(w1297, w1296, "veränderte Methode benutzen") -> (w1295:bool)
          n335 = case shown="True" "Methode speichern" {
            tunnel: w1293 -> [_ w1318]
            tunnel: w1300 -> [w1311 w1320]
            tunnel: w1299 -> [_ w1319]
            tunnel: [w1311 w1313] -> w1291
            frame False {
            }
            frame True {
              n336 = Replace Array Subset(array=w1320, new element=w1318, index=w1319) -> (w1313:T13)
              n337 = property on="Methode speichern" class="Bool (strict)"("Value"=FALSE ("Methode speichern")) -> ()  [unwired: 2 in, 2 out]
              n338 = Open/Create/Replace File(file path (use dialog)=path "c:/methoden.per" ("Dateipfad (Dialog verwenden)"), operation (0:open)=T14."replace" ("Operation (0:Öffnen)")) -> (refnum out=w1315:refnum<file>)  [unwired: 4 in, 2 out]
              n339 = Write to Binary File(file (use dialog)=w1315, data=w1313) -> (refnum out=w1312:refnum<file>)  [unwired: 4 in, 2 out]
              n340 = Close File(refnum=w1312) -> ()  [unwired: 1 in, 2 out]
            }
          }
          n341 = case shown="False" "veränderte Methode benutzen" {
            tunnel: w1293 -> [_ w1308]
            tunnel: [w1305 w1308] -> w1292
            tunnel: w1291 -> [w1307 _]
            frame False {
              n342 = local read "Methode"() -> (w1306:i32)
              n343 = Index Array(array=w1307, index=w1306) -> (element=w1305:T19)
            }
            frame True {
              n344 = flat-sequence {
                frame #0 {
                  n345 = call "Warten"("Count(mSec)"=u32 1100) -> ()  [unwired: 1 out]
                }
                frame #1 {
                  n346 = property on="veränderte Methode benutzen" class="Bool (strict)"("Value"=FALSE ("Methode verändern")) -> ()  [unwired: 2 in, 2 out]
                }
              }
            }
          }
        }
        n347 = Bundle(w993, w993, w993, w993) -> (w994:cluster{dbl[], dbl[], dbl[], dbl[]})  [unwired: 1 in]
        n348 = Bundle("ZyklusNummern"=w987, "ZeilennummernDIOs"=w1003, "ZwangsDIO?"=w991, "ZeilennummernHorst"=w1002, "ZwangsHorst?"=w992, "ZeileFPGABoolesch"=w1001, "ZwangsFPGABoolesch?"=w990, "ZeileFPGAPID"=w1000, "ZeileFPGAFixp"=w999, "ZeilePreMach1"=w998, "ZeilePreMach2"=w997, "ZeilennummerMPV"=w980, "ZeileMainMach1"=w924, "ZeileMainMach2"=w923, "ZwangsMPV?"=w908) -> (w996:T26)  [unwired: 1 in]
        n349 = call "arrayDoppelMoppel-11-15.vi"("verdoppeln"=i32[] [0, 1], "Traps/MachsKoeff2"=w912, "Traps/MachsKoeff1"=w916, "Traps/MachsKoeff0"=w922) -> ("Traps/MachsKoeff2"=w925:dbl[], "Traps/MachsKoeff1"=w926:dbl[], "Traps/MachsKoeff0"=w927:dbl[])  [unwired: 5 in]
        n350 = while {
          shift-right: [w1217] -> _
          shift-left: w994 -> [w1224]
          shift-right: [w1216] -> _
          shift-left: w994 -> [w1223]
          shift-right: [w1214] -> _
          shift-left: T17 {"Zyklus1"=0, "Zeitachse1"=0, "dargestellte Größe 1"=0, "Zyklus2"=0, "Zeitachse2"=0, "dargestellte Größe 2"=0} ("AnzeigeEinstellungen") -> [w1222]
          tunnel: w977 -> [w1192]
          shift-right: [w1188] -> _
          shift-left: w986 -> [w1187]
          shift-right: [w1183] -> _
          shift-left: w984 -> [w1185]
          shift-right: [w1172] -> _
          shift-left: w984 -> [w1184]
          shift-right: ["Detektor"] -> _
          shift-left: 0 ("Detektor") -> [w1181]
          tunnel: w905 -> [w1170]
          stop <- w1228 stop-if-true
          w1193 = 0.0 ("X-Achse.Bereich:Minimum")
          n351 = Unbundle(w1170) -> ("Modul1/AI sicherer Bereich"=w1163:dbl[][], "Modul2/AI sicherer Bereich"=w1148:dbl[][], "Modul3/AI sicherer Bereich"=w1139:dbl[][], "Traps/Machs sicherer Bereich"=w1130:dbl[][], w1122:dbl[][], "Metavariablen grüner Bereich"=w1113:dbl[][])
          n352 = call "Bis zum nächsten Vielfachen warten14"("Count(mSec)"=u32 1000) -> ()  [unwired: 1 out]
          n353 = global read "GVMWHorst.vi" "MWHorst"() -> (w1121:dbl[])
          "MWHorst" <- w1121
          n354 = case shown="0, Default" "Detektor" {
            tunnel: [w1238 w1250] -> w1183
            tunnel: w1192 -> [w1237 w1252]
            tunnel: "Detektor" -> [w1232 w1246]
            tunnel: [w1236 w1251] -> w1190
            tunnel: [w1235 w1249] -> w1188
            frame 0, Default {
              n355 = Increment(x=w1232) -> (x+1=w1233:i32)
              n356 = Increment(x=w1233) -> (x+1=w1231:i32)
              n357 = global read "GVChroms.vi" "ECD1Chrom"() -> (w1234:dbl[])
              n358 = global read "GVaktuelleTDMS.vi" "aktuelleTDMS-DateiECD1"() -> (w1235:refnum<k34>)
              n359 = Index Array(array=w1237, index=w1231) -> (element=w1236:dbl)
              n360 = Array Size(array=w1234) -> (size(s)=w1240:i32)
              n361 = for {
                N: w1240 -> [_]
                tunnel: [w1241] -> w1239 mode=indexing
                i -> [w1244]
                n362 = To Double Precision Float(number=w1244) -> (double precision float=w1243:dbl)
                n363 = Divide(x=w1243, y=10.0) -> (x/y=w1241:dbl)
              }
              n364 = Bundle(w1239, "ECD1Chrom"=w1234) -> (w1238:cluster{dbl[], "ECD1Chrom":dbl[]})  [unwired: 1 in]
            }
            frame 1 {
              n365 = Increment(x=w1246) -> (x+1=w1247:i32)
              n366 = Increment(x=w1247) -> (x+1=w1245:i32)
              n367 = global read "GVChroms.vi" "ECD2Chrom"() -> (w1248:dbl[])
              n368 = global read "GVaktuelleTDMS.vi" "aktuelleTDMS-DateiECD2"() -> (w1249:refnum<k34>)
              n369 = Index Array(array=w1252, index=w1245) -> (element=w1251:dbl)
              n370 = Array Size(array=w1248) -> (size(s)=w1254:i32)
              n371 = for {
                N: w1254 -> [_]
                tunnel: [w1255] -> w1253 mode=indexing
                i -> [w1258]
                n372 = To Double Precision Float(number=w1258) -> (double precision float=w1257:dbl)
                n373 = Divide(x=w1257, y=10.0) -> (x/y=w1255:dbl)
              }
              n374 = Bundle(w1253, "ECD2Chrom"=w1248) -> (w1250:cluster{dbl[], "ECD2Chrom":dbl[]})  [unwired: 1 in]
            }
          }
          n375 = Subtract(x="DetYMax", y="DetYMin") -> (x-y=w1198:dbl)
          n376 = Subtract(x="HK1YMax", y="HK1YMin") -> (x-y=w1208:dbl)
          n377 = Subtract(x="HK2YMax", y="HK2YMin") -> (x-y=w1203:dbl)
          n378 = Equal?(x="Detektor", y=w1181) -> (x = y?=w1180:bool)
          n379 = Index Array(array=w1163, index (col) #1=0 ("disabled index (col)"), index (col) #2=1 ("index (col)")) -> (element #1=w1160:dbl[], element #2=w1158:dbl[])  [unwired: 2 in]
          n380 = Index Array(array=w1148, index (col) #1=0 ("disabled index (col)"), index (col) #2=1 ("index (col)")) -> (element #1=w1152:dbl[], element #2=w1151:dbl[])  [unwired: 2 in]
          n381 = Index Array(array=w1130, index (col) #1=0 ("disabled index (col)"), index (col) #2=1 ("index (col)")) -> (element #1=w1134:dbl[], element #2=w1133:dbl[])  [unwired: 2 in]
          n382 = Index Array(array=w1122, index (col) #1=0 ("disabled index (col)"), index (col) #2=1 ("index (col)")) -> (element #1=w1126:dbl[], element #2=w1125:dbl[])  [unwired: 2 in]
          n383 = Index Array(array=w1139, index (col) #1=0 ("disabled index (col)"), index (col) #2=1 ("index (col)")) -> (element #1=w1143:dbl[], element #2=w1142:dbl[])  [unwired: 2 in]
          n384 = Index Array(array=w1113, index (col) #1=0 ("disabled index (col)"), index (col) #2=1 ("index (col)")) -> (element #1=w1117:dbl[], element #2=w1116:dbl[])  [unwired: 2 in]
          n385 = global read "GVMethodenwechsel.vi" "Methodenwechsel?"() -> (w1226:bool)
          n386 = global read "GVZeitenZyklen.vi" "ZyklusNummern"() -> (w1195:i32[])
          "ZyklusNummern" <- w1195
          n387 = global read "gvbooleschRT.vi" "global stop RT"() -> (w1227:bool)
          n388 = global read "GVMetavariablen.vi" "Metavariablen"() -> (w1112:dbl[])
          "Metavariablen" <- w1112
          n389 = global read "GVVentilposition.vi" "Ventilposition"() -> (→"Ventilposition":i32)
          n390 = global read "GVZeitenZyklen.vi" "ZyklusNummernGesamt"() -> (→"ZyklusNummernGesamt":i32[])
          n391 = Divide(x=w1198, y=20.0) -> (x/y=w1196:dbl)
          n392 = Divide(x=w1208, y=10.0) -> (x/y=w1206:dbl)
          n393 = Divide(x=w1203, y=10.0) -> (x/y=w1201:dbl)
          n394 = local read "veränderte Methode benutzen"() -> (w1225:bool)
          n395 = Or(x=w1226, y=w1227) -> (x .or. y?=w1229:bool)
          n396 = Greater Or Equal?(x=w1121, y=w1126) -> (x >= y?=w1124:bool[])
          n397 = Less Or Equal?(x=w1121, y=w1125) -> (x <= y?=w1123:bool[])
          n398 = Greater Or Equal?(x=w1112, y=w1117) -> (x >= y?=w1115:bool[])
          n399 = Less Or Equal?(x=w1112, y=w1116) -> (x <= y?=w1114:bool[])
          n400 = global read "GVHK1Hz.vi" "Mod1Mod2Mod3/AITrapsMachs1Hz"() -> (w1108:dbl[])
          n401 = And(x=w1124, y=w1123) -> (x .and. y?=→"HorstOK?":bool[])
          n402 = And(x=w1115, y=w1114) -> (x .and. y?=→"MVOK?":bool[])
          n403 = Or(x=w1229, y=w1225) -> (x .or. y?=w1228:bool)
          n404 = global read "GVZeitenZyklen.vi" "Big Ben, Methodenzeit, Zykluszeit0, Zykluszeit1, Zykluszeit2A, Zykluszeit2B"() -> (w1175:dbl[])
          n405 = Array Subset(array=w1108, index=0 ("Index"), length=32 ("Länge")) -> (w1159:dbl[])
          "AIs1" <- w1159
          n406 = Array Subset(array=w1108, index=32 ("Index"), length=32 ("Länge")) -> (w1147:dbl[])
          "AIs2" <- w1147
          n407 = Array Subset(array=w1108, index=96 ("Index"), length=6 ("Länge")) -> (w1107:dbl[])
          "schnelle Heizungen" <- w1107
          n408 = Array Subset(array=w1108, index=64 ("Index"), length=32 ("Länge")) -> (w1138:dbl[])
          "AIs3" <- w1138
          n409 = Greater Or Equal?(x=w1107, y=w1134) -> (x >= y?=w1132:bool[])
          n410 = Less Or Equal?(x=w1107, y=w1133) -> (x <= y?=w1131:bool[])
          n411 = Greater Or Equal?(x=w1159, y=w1160) -> (x >= y?=w1157:bool[])
          n412 = Less Or Equal?(x=w1159, y=w1158) -> (x <= y?=w1156:bool[])
          n413 = Greater Or Equal?(x=w1147, y=w1152) -> (x >= y?=w1150:bool[])
          n414 = Less Or Equal?(x=w1147, y=w1151) -> (x <= y?=w1149:bool[])
          n415 = And(x=w1132, y=w1131) -> (x .and. y?=→"SHOK?":bool[])
          n416 = Greater Or Equal?(x=w1138, y=w1143) -> (x >= y?=w1141:bool[])
          n417 = Less Or Equal?(x=w1138, y=w1142) -> (x <= y?=w1140:bool[])
          n418 = And(x=w1157, y=w1156) -> (x .and. y?=→"AIs1OK?":bool[])
          n419 = And(x=w1150, y=w1149) -> (x .and. y?=→"AIs2OK?":bool[])
          n420 = And(x=w1141, y=w1140) -> (x .and. y?=→"AIs3OK?":bool[])
          n421 = To Long Integer(number=w1175) -> (32bit integer=→"Big Ben, Methodenzeit, Zykluszeit0, Zykluszeit1, Zykluszeit2A, Zykluszeit2B":i32[])
          n422 = Equal?(x=w1188, y=w1187) -> (x = y?=w1186:bool)
          n423 = call "AnzeigeGV.vi"("veränderte Methode benutzen"=w1225, "Zykluslängen [s]"=w1192, "Cluster1"=w1224, "Big Ben, Methodenzeit, Zykluszeit0, Zykluszeit1, Zykluszeit2A, Zykluszeit2B"=w1175, "Zyklusnummern 0, 1, 2A, 2B"=w1195, "Cluster2"=w1223, "AnzeigeEinstellungen"=w1222, "dargestellte Größe 1"="dargestellte Größe 1", "Zeitachse1"="Zeitachse1", "dargestellte Größe 2"="dargestellte Größe 2", "Zeitachse2"="Zeitachse2") -> ("Anzeige2"=→"Housekeeping2":cluster{dbl[], dbl[]}, "Cluster1"=w1217:cluster{dbl[], dbl[], dbl[], dbl[]}, "x1Inkr"=w1212:dbl, "Cluster2"=w1216:cluster{dbl[], dbl[], dbl[], dbl[]}, "Anzeige1"=→"Housekeeping1":cluster{dbl[], dbl[]}, "AnzeigeEinstellungen"=w1214:T17, "x2Max"=w1176:dbl, "x2Inkr"=w1211:dbl, "x1Max"=w1177:dbl)  [unwired: 8 in]
          n424 = Divide(x=w1190, y=20.0) -> (x/y=w1191:dbl)
          n425 = property on="Detektor 2" class="XYGraph (strict)"("XScale.Minimum"=w1193, "XScale.Maximum"=w1190, "XScale.Increment"=w1191, "YScale.Minimum"="DetYMin", "YScale.Maximum"="DetYMax", "YScale.Increment"=w1196) -> ()  [unwired: 2 in, 2 out]
          n426 = property on="Housekeeping1" class="XYGraph (strict)"("XScale.Minimum"=w1193, "XScale.Maximum"=w1177, "XScale.Increment"=w1212, "YScale.Minimum"="HK1YMin", "YScale.Maximum"="HK1YMax", "YScale.Increment"=w1206) -> ()  [unwired: 2 in, 2 out]
          n427 = property on="Housekeeping2" class="XYGraph (strict)"("XScale.Minimum"=w1193, "XScale.Maximum"=w1176, "XScale.Increment"=w1211, "YScale.Minimum"="HK2YMin", "YScale.Maximum"="HK2YMax", "YScale.Increment"=w1201) -> ()  [unwired: 2 in, 2 out]
          n428 = Select(t=w1184, s=w1186, f=w1185) -> (s? t:f=w1179:cluster{dbl[], dbl[]})
          n429 = Select(t=w1179, s=w1180, f=cluster{dbl[], dbl[]} {[], []} ("s? t:f")) -> (s? t:f=w1172:cluster{dbl[], dbl[]})
          n430 = Build Array(w1183, w1172) -> (→"Detektor 2":cluster{dbl[], "ECD2Chrom":dbl[]}[])
        }
        n431 = while "ZyklusSteuerung" {
          tunnel: w1021 -> [w1269]
          tunnel: w1022 -> [w1259]
          shift-right: [w1268] -> _
          shift-left: w996 -> [w1262]
          tunnel: w1004 -> [w1266]
          tunnel: w927 -> [w1265]
          tunnel: w926 -> [w1264]
          tunnel: w925 -> [w1263]
          tunnel: w910 -> [w1267]
          shift-right: [w1261] -> _
          shift-left: errorcluster {"status"=FALSE, "code"=0, "source"=""} ("error out") -> [w1260]
          stop <- w1271 stop-if-true
          n432 = call "Bis zum nächsten Vielfachen warten11"("Count(mSec)"=u32 100) -> ()  [unwired: 1 out]
          n433 = global read "GVMethodenwechsel.vi" "Methodenwechsel?"() -> (w1274:bool)
          n434 = global read "gvbooleschRT.vi" "global stop RT"() -> (w1273:bool)
          n435 = local read "veränderte Methode benutzen"() -> (w1272:bool)
          n436 = call "ZyklussteuerungGV-01-17.vi"("Traps/MachKoeff0"=w1265, "DIOsNummern"=w1269, "error in"=w1260, "Traps/MachKoeff1"=w1264, "ServosWarmHigh (us)KaltHigh(us)"="ServosWarmHigh (us)KaltHigh(us)", "Traps/MachKoeff2"=w1263, "Schieberegister"=w1262, "Zeitpunkte/Setpoints"=w1266, "FPGA VI Reference In"=w1259, "MachKoeffs"=w1267) -> ("Schieberegister"=w1268:T27, "error out"=w1261:errorcluster)  [unwired: 4 in]
          "Zyklus" <- w1261
          n437 = Compound Arithmetic op=OR(w1274, w1273, w1272) -> (w1271:bool)
        }
        n438 = global read "GVZeitenZyklen.vi" "Big Ben, Methodenzeit, Zykluszeit0, Zykluszeit1, Zykluszeit2A, Zykluszeit2B"() -> (w983:dbl[])
        n439 = Index Array(array=w983, index=3 ("Index")) -> (element=w981:dbl)
        n440 = while {
          tunnel: w1025 -> [w1052]
          tunnel: w1024 -> [w1051]
          tunnel: w946 -> [w1066]
          shift-right: [w1067] -> w1018
          shift-left: w1023 -> [w1068]
          tunnel: w943 -> [w1062]
          tunnel: w942 -> [w1056]
          shift-right: [w1053] -> _
          shift-left: w981 -> [w1057]
          stop <- w1069 stop-if-true
          n441 = Less?(x=w1057, y=w1062) -> (x < y?=w1060:bool)
          n442 = Less?(x=w1057, y=w1056) -> (x < y?=w1058:bool)
          n443 = call "Bis zum nächsten Vielfachen warten13"("Count(mSec)"=u32 100 ("Zu wartende ms")) -> ()  [unwired: 1 out]
          n444 = global read "GVMethodenwechsel.vi" "Methodenwechsel?"() -> (w1071:bool)
          n445 = global read "gvbooleschRT.vi" "global stop RT"() -> (w1072:bool)
          n446 = local read "veränderte Methode benutzen"() -> (w1070:bool)
          n447 = Compound Arithmetic op=OR(w1072, w1071, w1070) -> (w1069:bool)
          n448 = global read "GVZeitenZyklen.vi" "Big Ben, Methodenzeit, Zykluszeit0, Zykluszeit1, Zykluszeit2A, Zykluszeit2B"() -> (w1064:dbl[])
          n449 = Index Array(array=w1064, index=3 ("Index")) -> (element=w1053:dbl)
          n450 = Greater Or Equal?(x=w1053, y=w1062) -> (x >= y?=w1061:bool)
          n451 = Greater Or Equal?(x=w1053, y=w1056) -> (x >= y?=w1059:bool)
          n452 = And(x=w1059, y=w1058) -> (x .and. y?=w1055:bool)
          n453 = And(x=w1061, y=w1060) -> (x .and. y?=w1050:bool)
          n454 = Or(x=w1050, y=w1055) -> (x .or. y?=w1054:bool)
          n455 = And(x=w1066, y=w1054) -> (x .and. y?=w1065:bool)
          n456 = case shown="True" w1065 {
            tunnel: w1068 -> [w1074 w1075]
            tunnel: [w1074 w1079] -> w1067
            tunnel: w1052 -> [_ w1078]
            tunnel: w1051 -> [_ w1077]
            tunnel: w1050 -> [_ w1076]
            frame False {
            }
            frame True {
              n457 = call "MSDateienSchicken12-15.vi"("MSNummer"=w1075, "MSa?"=w1076, "Dateipfad:fromcriordy"=w1077, "Dateipfad:fromcriocmd"=w1078) -> ()  [unwired: 1 in]
              n458 = Increment(x=w1075) -> (x+1=w1079:i32)
            }
          }
        }
      }
      n459 = Add Array Elements(numeric array=w478) -> (sum=w488:i32)
      n460 = Index Array(array=w478, index #1=0 ("Index"), index #2=1 ("Index")) -> (element #1=w499:i32, element #2=w497:i32)
      n461 = Split 1D Array(array=w477, index=w499) -> (first subarray=w503:dbl[], second subarray=w507:dbl[])
      n462 = Split 1D Array(array=w475, index=w499) -> (first subarray=w506:string[], second subarray=w508:string[])
      n463 = Split 1D Array(array=w476, index=w499) -> (first subarray=w496:string[], second subarray=w498:string[])
      n464 = Initialize Array(-1.0 ("Element"), w488) -> (w473:dbl[])
      n465 = Split 1D Array(array=w508, index=w497) -> (first subarray=w505:string[], second subarray=w504:string[])
      n466 = Split 1D Array(array=w507, index=w497) -> (first subarray=w502:dbl[], second subarray=w501:dbl[])
      n467 = Split 1D Array(array=w498, index=w497) -> (first subarray=w495:string[], second subarray=w494:string[])
      n468 = Bundle(w506, w505, w504, w503, w502, w501) -> (w500:T28)  [unwired: 1 in]
      n469 = Bundle(w496, w495, w494) -> (w493:cluster{string[], string[], string[]})  [unwired: 1 in]
      n470 = Initialize Array(0.0, 8 ("Dimension")) -> (w423:dbl[])
      n471 = Bundle(w492, w492, w492) -> (w491:cluster{i32, i32, i32})  [unwired: 1 in]
      n472 = Initialize Array("x", 8 ("Dimension")) -> (w428:string[])
      n473 = case shown="True" TRUE ("SerielleKomm.") {
        tunnel: bool[] [TRUE, TRUE, TRUE, TRUE, TRUE, TRUE, TRUE, TRUE] -> [_ w565]
        tunnel: w428 -> [_ w564]
        tunnel: w500 -> [_ w563]
        tunnel: w499 -> [_ w562]
        tunnel: w497 -> [_ w561]
        tunnel: w493 -> [_ w560]
        tunnel: w491 -> [_ w559]
        tunnel: w490 -> [_ w558]
        tunnel: w477 -> [_ w557]
        tunnel: w474 -> [_ w556]
        tunnel: w473 -> [_ w555]
        tunnel: w472 -> [_ w552]
        tunnel: w451 -> [_ w554]
        tunnel: w423 -> [_ w553]
        tunnel: w422 -> [_ w551]
        frame False {
        }
        frame True {
          n474 = while {
            tunnel: w552 -> [w579]
            tunnel: w551 -> [w578]
            shift-right: [w577] -> _
            shift-left: errorcluster {"status"=FALSE, "code"=0, "source"=""} ("error out") -> [w576]
            stop <- w580 stop-if-true
            n475 = call "Warten6"("Count(mSec)"=u32 500) -> ()  [unwired: 1 out]
            n476 = global read "gvbooleschRT.vi" "global stop RT"() -> (w580:bool)
            n477 = case shown="True" "NeuerRefstrom" {
              tunnel: w578 -> [w582 _]
              tunnel: [w581 w591] -> w571
              tunnel: [w581 w594] -> w567
              frame False {
                n478 = String To Byte Array(string=w582) -> (unsigned byte array=w581:u8[])
              }
              frame True {
                n479 = local write "NeuerRefstrom"(FALSE ("NeuerRefstrom")) -> ()
                n480 = Number To Decimal String(number="RefStromECD1", width (-)=i16 4) -> (decimal integer string=w586:string)
                n481 = Number To Decimal String(number="RefStromECD2", width (-)=i16 4) -> (decimal integer string=w583:string)
                n482 = Concatenate Strings("?SE0,SETP," ("string"), w586, "\r\n") -> (w595:string)
                n483 = Concatenate Strings("?SE0,SETP," ("string"), w583, "\r\n") -> (w592:string)
                n484 = String To Byte Array(string=w595) -> (unsigned byte array=w594:u8[])
                n485 = String To Byte Array(string=w592) -> (unsigned byte array=w591:u8[])
              }
            }
            n486 = Join Numbers(hi=w567, lo=u8 5) -> ((hi.lo)=w573:u16[])
            n487 = Join Numbers(hi=w571, lo=u8 6) -> ((hi.lo)=w569:u16[])
            n488 = xnode "Invoke Method"("FPGA VI Reference In"=w579, "error in"=w576, "Data"=w573) -> ("FPGA VI Reference Out"=w572:refnum<k20>, "error out"=w568:errorcluster)  [unwired: 1 in, 1 out]
            n489 = xnode "Invoke Method"("FPGA VI Reference In"=w572, "error in"=w568, "Data"=w569) -> ("error out"=w577:errorcluster)  [unwired: 1 in, 2 out]
            "FIFOwriteRS485" <- w577
          }
          n490 = while {
            shift-right: [w735] -> _
            shift-left: w565 -> [w750]
            shift-right: [w754] -> _
            shift-left: w555 -> [w760]
            tunnel: w552 -> [w749]
            shift-right: [w736] -> _
            shift-left: w564 -> [w738]
            tunnel: w556 -> [w740]
            tunnel: w557 -> [w737]
            shift-right: [w741] -> _
            shift-left: w558 -> [w756]
            tunnel: w562 -> [w758]
            tunnel: w561 -> [w759]
            tunnel: w563 -> [w761]
            tunnel: w560 -> [w743]
            shift-right: [w742] -> _
            shift-left: w559 -> [w744]
            shift-right: [w747] -> _
            shift-left: w554 -> [w748]
            shift-right: [w751] -> _
            shift-left: w553 -> [w752]
            shift-right: [w732] -> _
            shift-left: errorcluster {"status"=FALSE, "code"=0, "source"=""} ("error out") -> [w731]
            stop <- w755 stop-if-true
            n491 = for {
              tunnel: w750 -> [w765] mode=indexing
              tunnel: w752 -> [w762] mode=indexing
              tunnel: [w769] -> w751 mode=indexing
              tunnel: [w766] -> w745 mode=indexing
              n492 = global read "GVZeitenZyklen.vi" "Big Ben, Methodenzeit, Zykluszeit0, Zykluszeit1, Zykluszeit2A, Zykluszeit2B"() -> (w772:dbl[])
              n493 = Index Array(array=w772, index=0 ("Index")) -> (element=w770:dbl)
              n494 = Subtract(x=w770, y=w762) -> (x-y=w768:dbl)
              n495 = Greater?(x=w768, y=0.1) -> (0:w764:bool)
              n496 = Or(x=w765, y=w764) -> (x .or. y?=w763:bool)
              n497 = Select(t=w764, s=w764, f=w765) -> (s? t:f=w766:bool)
              n498 = Select(t=w770, s=w763, f=w762) -> (s? t:f=w769:dbl)
            }
            n499 = call "MPVSenden-01-17.vi"("Ventilposition"=w748, "error in"=w731, "FPGA VI Reference In"=w749) -> ("Ventilposition"=w747:i32, "error out"=w734:errorcluster, "FPGA VI Reference Out"=w730:refnum<k20>)
            n500 = call "Warten3"("Count(mSec)"=u32 50) -> ()  [unwired: 1 out]
            n501 = global read "GVHorstSP.vi" "HorstSP"() -> (w754:dbl[])
            n502 = global read "gvbooleschRT.vi" "global stop RT"() -> (w755:bool)
            n503 = Not Equal?(x=w754, y=w760) -> (x != y?=w757:bool)
            n504 = call "NeueSP.vi"("Anzahl2"=w759, "Anzahl1"=w758, "AlteSP"=w760, 7:"NeueSP"=w754, "BefehleCluster"=w756, 10:"NeueSP"=w757, "ClusterFest"=w761) -> ("BefehleCluster"=w746:T29)  [unwired: 4 in]
            n505 = call "Senden-01-17.vi"("error in"=w734, "BefehlsCluster"=w746, "AbfragenCluster"=w743, "Abfragenr.Cluster"=w744, "Senden?"=w745, "FPGA VI Reference In"=w730) -> ("BefehlsCluster"=w741:T29, "error out"=w733:errorcluster, "Senden?"=w739:bool[], "Abfragenr.Cluster"=w742:cluster{i32, i32, i32})  [unwired: 1 in]
            n506 = call "SeriellRead-01-17.vi"("SkalierungsfaktorHorst"=w737, "VorwortHorst"=w740, "error in"=w733, "Zwischenspeicher"=w738, "Senden?"=w739, "FPGA VI Reference In"=w730) -> ("Senden?"=w735:bool[], "Zwischenspeicher"=w736:string[], "error out"=w732:errorcluster)  [unwired: 3 in]
            "SerielleKomm." <- w732
          }
        }
      }
    }
    frame #2 {
      n507 = xnode "Read/Write Control"("FPGA VI Reference In"=w1355, "global stop"=TRUE) -> ("FPGA VI Reference Out"=w1354:refnum<k20>)  [unwired: 1 in, 1 out]
      n508 = xnode "Close FPGA VI Reference"("FPGA VI Reference In"=w1354) -> ()  [unwired: 1 in, 1 out]
    }
    frame #3 {
    }
    frame #4 {
    }
  }
